vi "3.0.0_Power_Tunings & AW_Performance_Test_ECO_&_BOOST.vi"(6 ".bat":T1={"getVersion"="Getting Software Version.bat", "Start Test mode"="Start Test Mode.bat", "Start camera test mode"="Start camera test mode.bat", "get one RAW Image"="Get one image.bat", "Stop camera test mode"="Stop camera test mode.bat", "Stop Test Mode"="Stop Test Mode.bat", "Get image reflection"="Get image reflection.bat", "Get image uniformity andFlash LED brightness"="Get image uniformity andFlash LED brightness.bat", "Disable flash LED"="Disable flash LED.bat", "Enable flash LED"="Enable flash LED.bat", "Software Reset"="Software Reset.bat", "Tune Flash LED brightness"="Tune Flash LED brightness.bat", "Start Camera calibration"="Start Camera calibration.bat", "Verify OBC Setting"="Verify OBC Setting.bat"}, 7 "Data in":T2, 8 "error in (no error)":errorcluster, 9 "AllControls In":T3, 11 "Message Queue out":T4) -> (0 "error out":errorcluster, 1 "Flow":string, 3 "Message Queue Out":T4, 5 "Data out":T2)   [LabVIEW 2017]
uses:
  Depends/AMC/subVIs/TypeDefs/amc_Message Queue.ctl
  Depends/AMC/subVIs/TypeDefs/amc_Message.ctl
  Depends/Tools/Keyed Array/Tools_KeyedArray KeyedArray.ctl
  Ctrls/AllControls.ctl
  Ctrls/CSV_Data.ctl
  Ctrls/NFC.bat
panel:
  out "Unifority_Flag":bool
  out "Reflect_Flag":bool
  in  "Numeric 2":i32
  in  "Numeric":i32
types:
  T1 = typedef "NFC.bat" = cluster{"getVersion":string, "Start Test mode":string, "Start camera test mode":string, "get one RAW Image":string, "Stop camera test mode":string, "Stop Test Mode":string, "Get image reflection":string, "Get image uniformity andFlash LED brightness":string, "Disable flash LED":string, "Enable flash LED":string, "Software Reset":string, "Tune Flash LED brightness":string, "Start Camera calibration":string, "Verify OBC Setting":string}
  T2 = typedef "CSV_Data.ctl" = cluster{"Version":cluster{"SC_Version":string, "VP_Version":string}, "SN":string, "Table":string[][], "Count":cluster{"Total":i32, "OK":i32, "NG":i32, "Yield":dbl}, "Start Time":timestamp, "daemon reference":refnum<k5>, "CT":dbl, "Config":string[][], "OK/NG":bool, "Station ID":string, "MES DDM SN":string, "MES PCBA SN":string, "Retest":string, "Lux":string, "VOT":cluster{"Initial brightness":string, "Mean uniformity":string, "Uniformity_Deviation":string, "Adjusted brightness":string, "Mean_Adjusted":string, "Deviation_Adjusted":string, "Reflection":string, "Result":bool}, "SKU":string, "Plate_Diameter":string, "Alarm":string}
  T3 = typedef "AllControls.ctl" = cluster{"MainVI":refnum<vi>, "AlarmInfo":refnum<vi>, "Log":refnum<vi>, "Current CT":refnum<vi>, "ProductID":refnum<vi>, "Device state":refnum<vi>, "MES":refnum<vi>, "mode":refnum<vi>, "TestInfo":refnum<vi>, "SubPnl":refnum<vi>, "Table":refnum<vi>, "MES bool":refnum<vi>, "TestMode":refnum<vi>, "Recipe":refnum<vi>, "Fail resume":refnum<vi>, "LogIn":refnum<vi>, "Start":refnum<vi>, "Maintenance":refnum<vi>, "Stop":refnum<vi>, "Exit":refnum<vi>}
  T4 = typedef "amc_Message Queue.ctl" = refnum<queue>
  T5 = cluster{"getVersion":string, "Start Test mode":string, "Start camera test mode P1":string, "get one RAW Image":string, "Start camera test mode P0":string, "Stop Test Mode":string, "Stop Camera":string}
  T6 = typedef "HD Config.ctl" = cluster{" PC":cluster{"PC Address":u8[], "PC Port":i32}, "FCO":cluster{"COM":refnum<visa-resource-name>, "Baudrate":u32}, "DC Power ":cluster{"COM":refnum<visa-resource-name>, "Baudrate":u32}, "PW3336":cluster{"COM":refnum<visa-resource-name>, "Baudrate":u32}, "Lefoo":cluster{"COM":refnum<visa-resource-name>, "Baudrate":u32}, "Tempt&Hum":cluster{"COM":refnum<visa-resource-name>, "Baudrate":u32}, "DIPC":cluster{"COM":refnum<visa-resource-name>}, "Daemon":cluster{"IP Address":string, "Port":u16, "Retry":u16}, "NFC_Cmd":cluster{"COM":refnum<visa-resource-name>, "Baudrate":u32}, "Fail_resume_mode":bool, "GRR":bool, "NFC _Serial":cluster{"COM":refnum<visa-resource-name>, "Baudrate":u32}}
  T7 = typedef "Position Config.ctl" = cluster{"Black":dbl, "White":dbl, "Black1":dbl, "White1":dbl}
  T8 = typedef "TesterInfo.ctl" = cluster{"Station Name":string, "Station Code":string, "ES NO.":string, "Tester ID":string, "PassMark Revision":string, "Rig ID":string, "682_Tool_Repeat":string, "Project Name":string, "FFTesterPath":path, "Enable_User":bool, "Mode":enum16{"682"}, "Fail_resume_mode":bool}
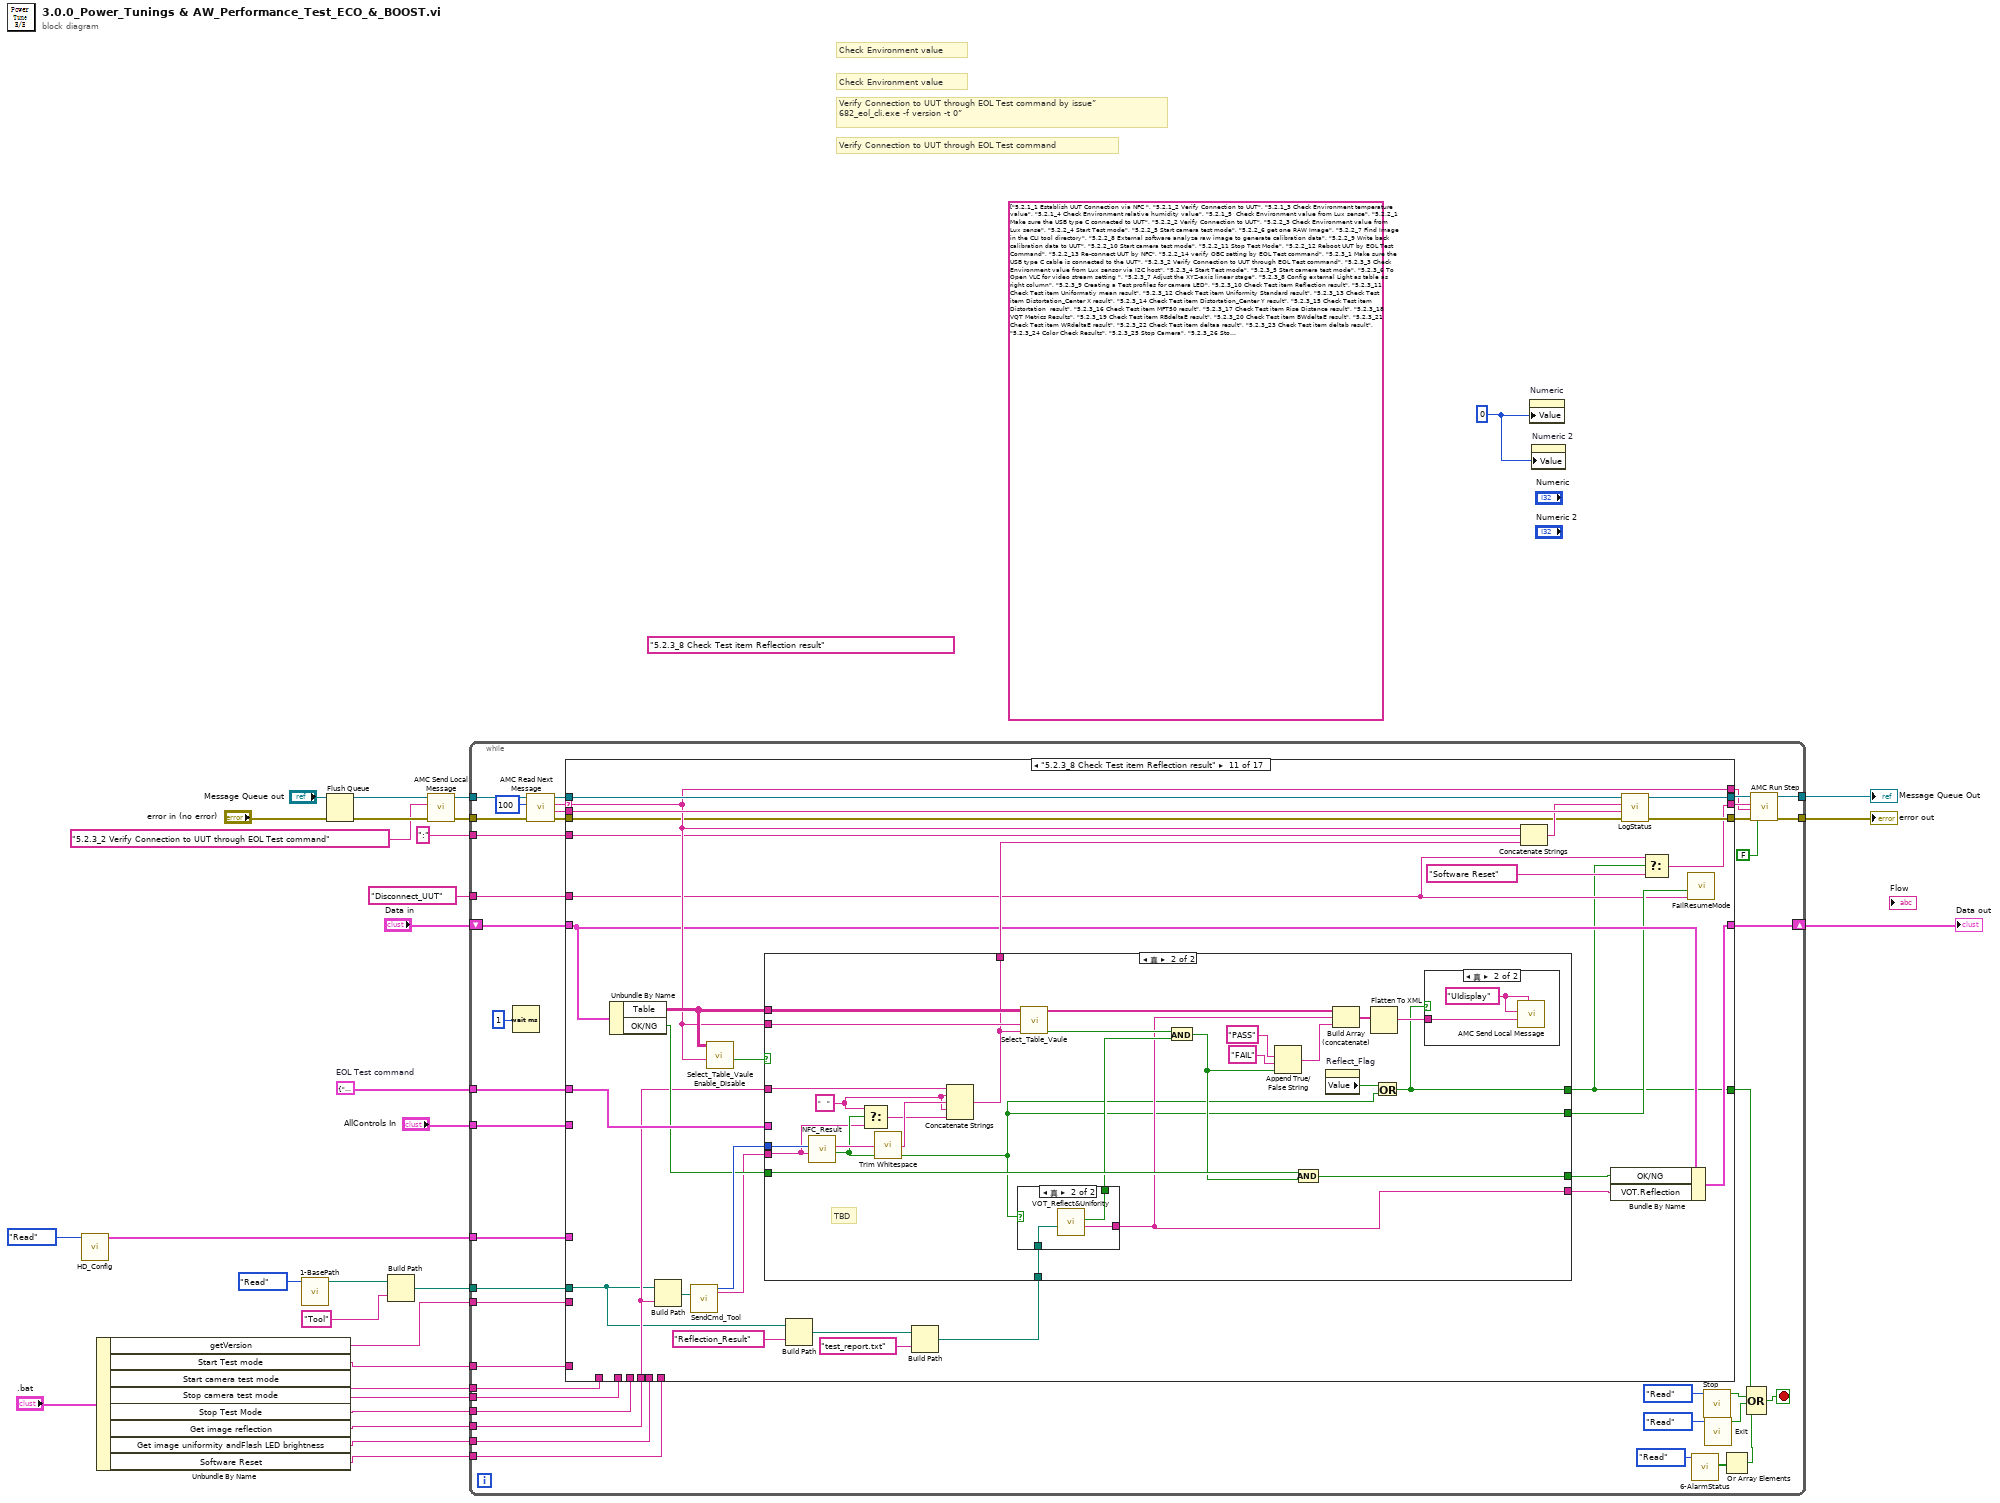
[diagram p0: block diagram]
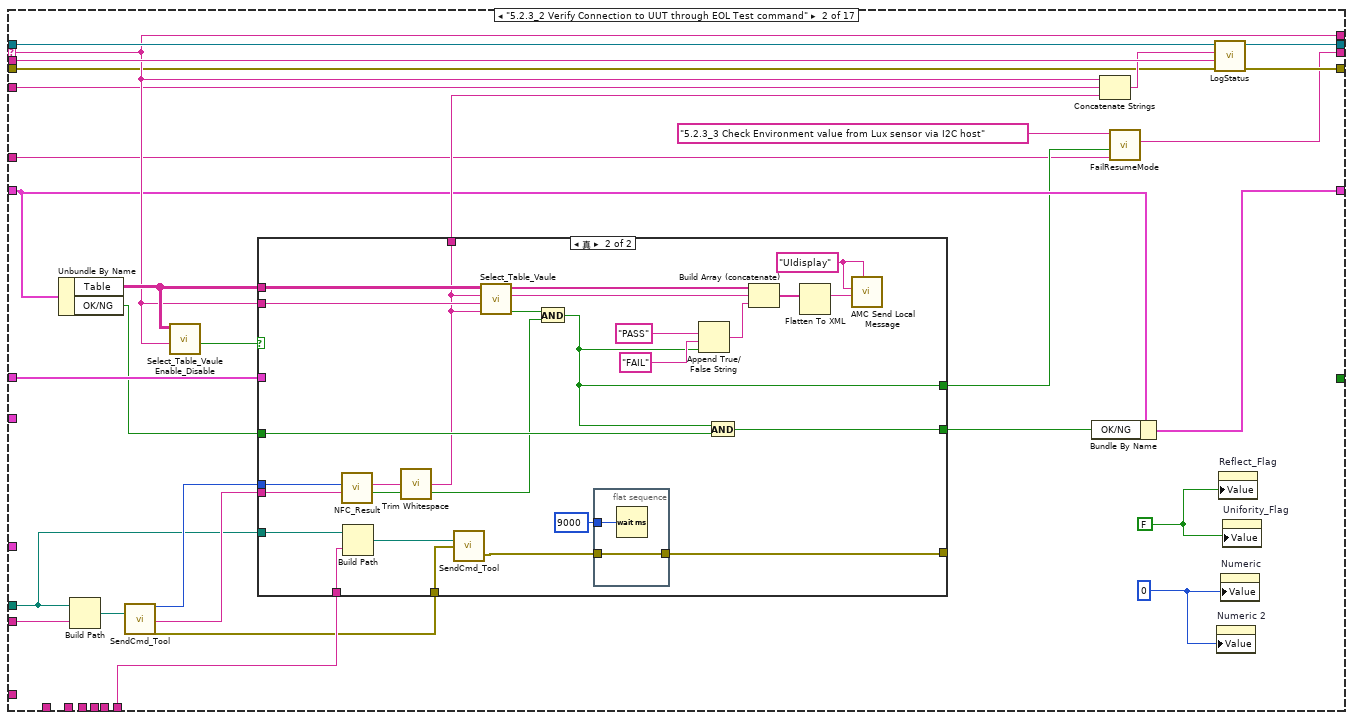
[diagram p3: hidden frame]
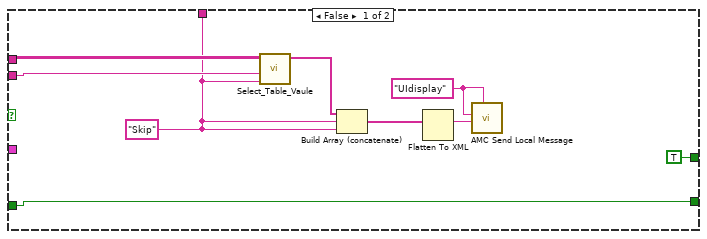
[diagram p4: hidden frame]
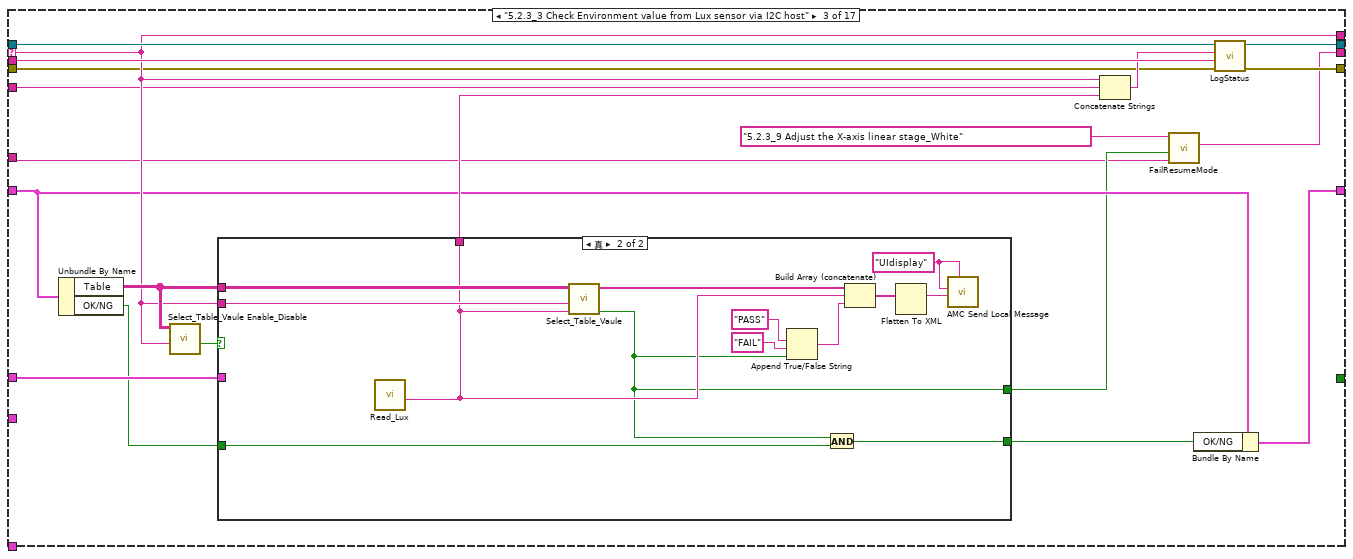
[diagram p5: hidden frame]
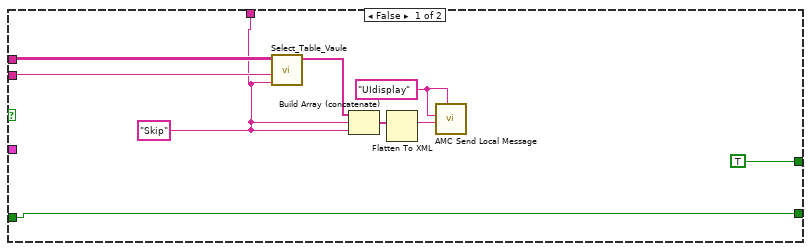
[diagram p6: hidden frame]
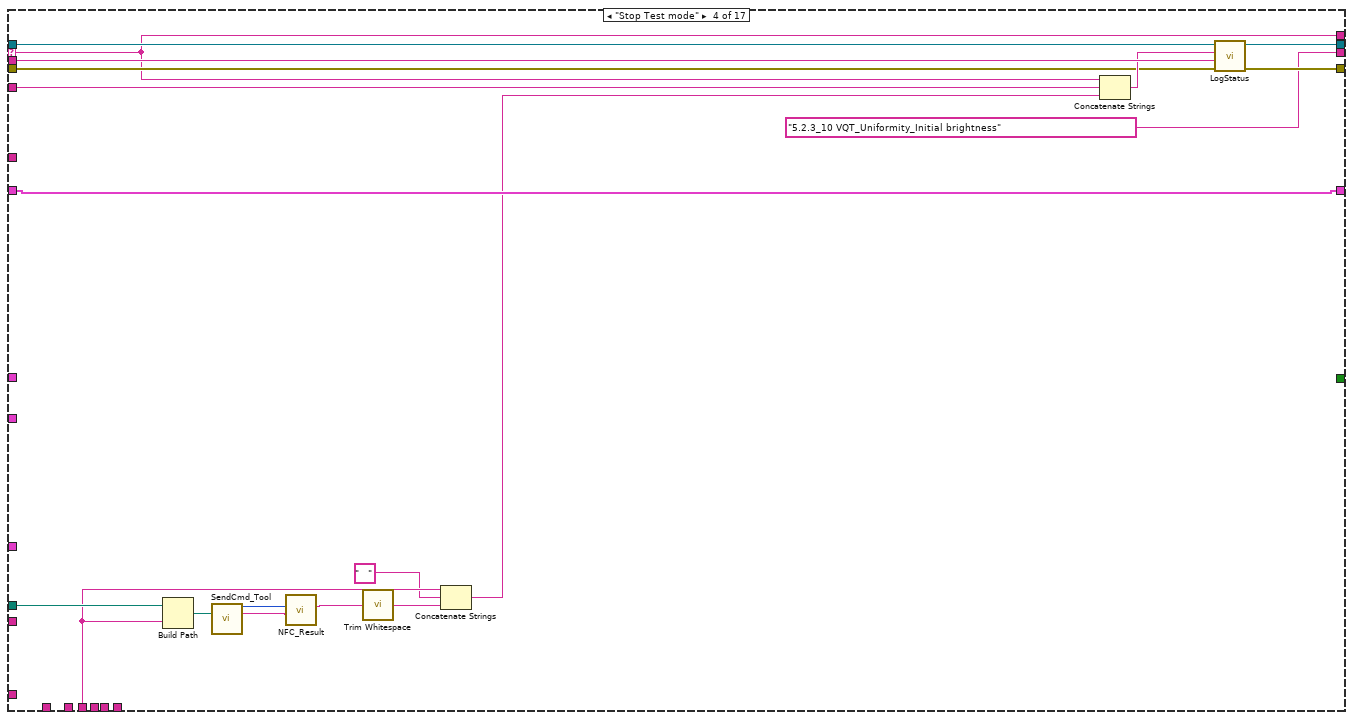
[diagram p7: hidden frame]
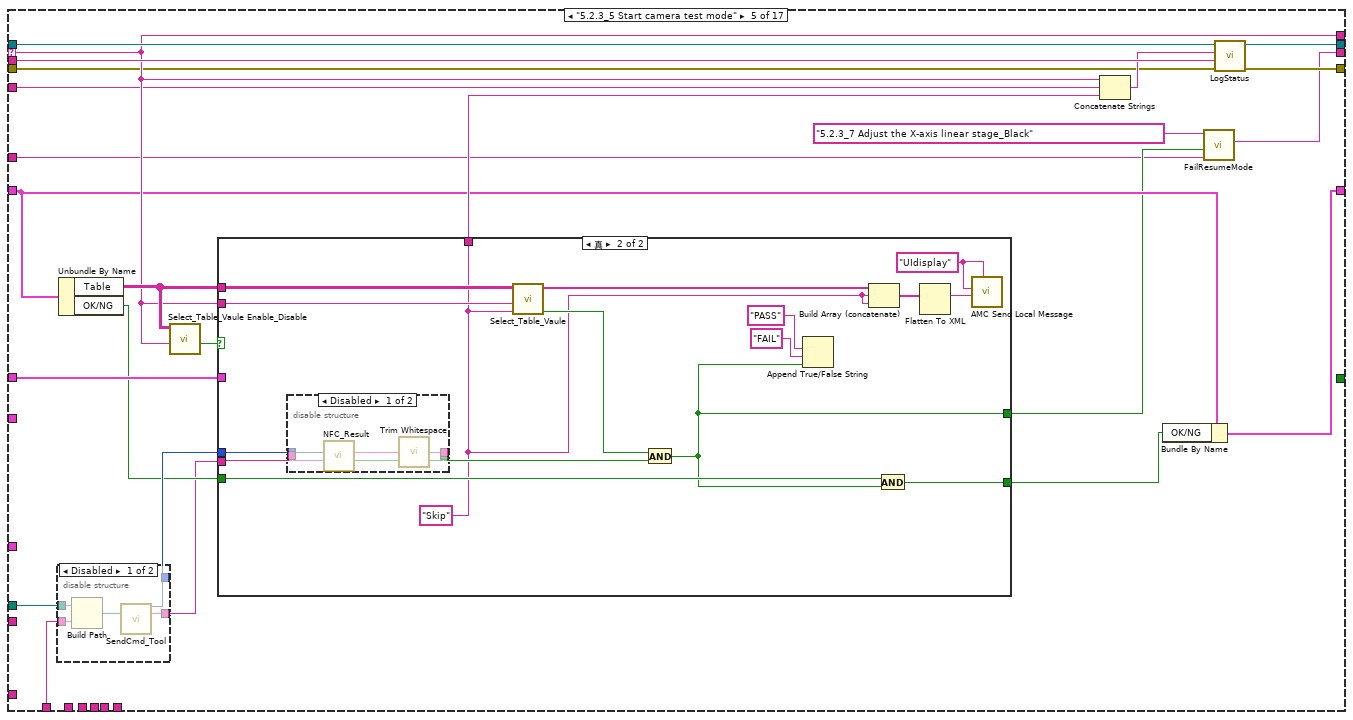
[diagram p8: hidden frame]
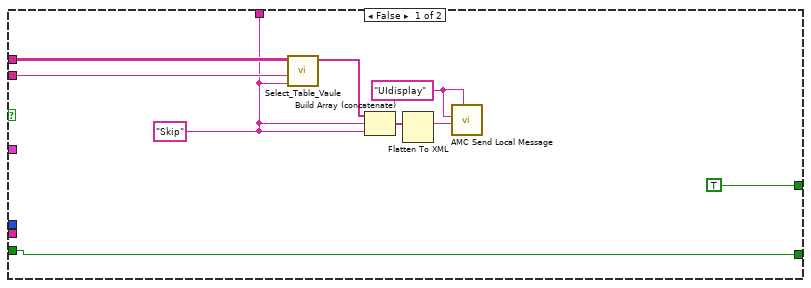
[diagram p10: hidden frame]
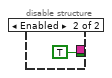
[diagram p11: hidden frame]
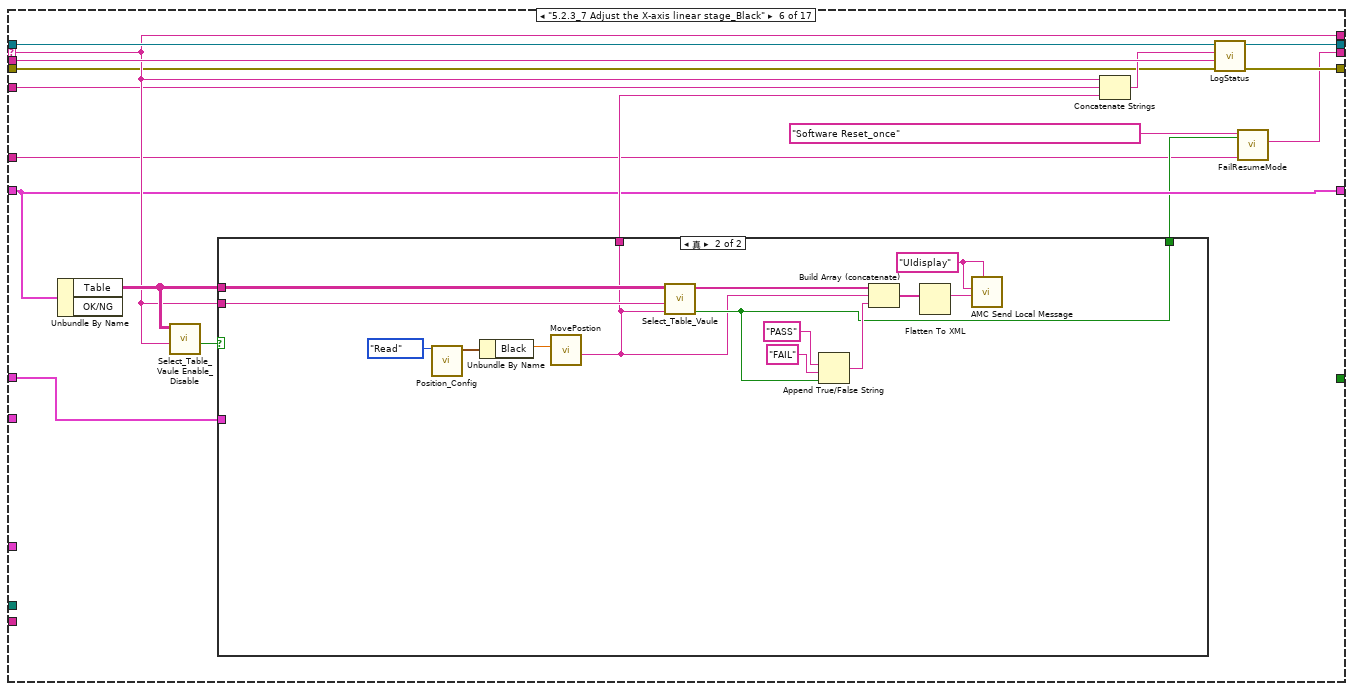
[diagram p12: hidden frame]
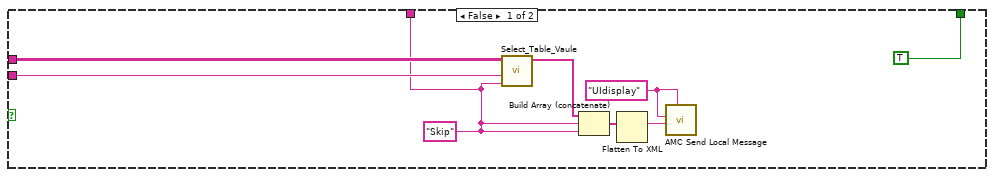
[diagram p13: hidden frame]
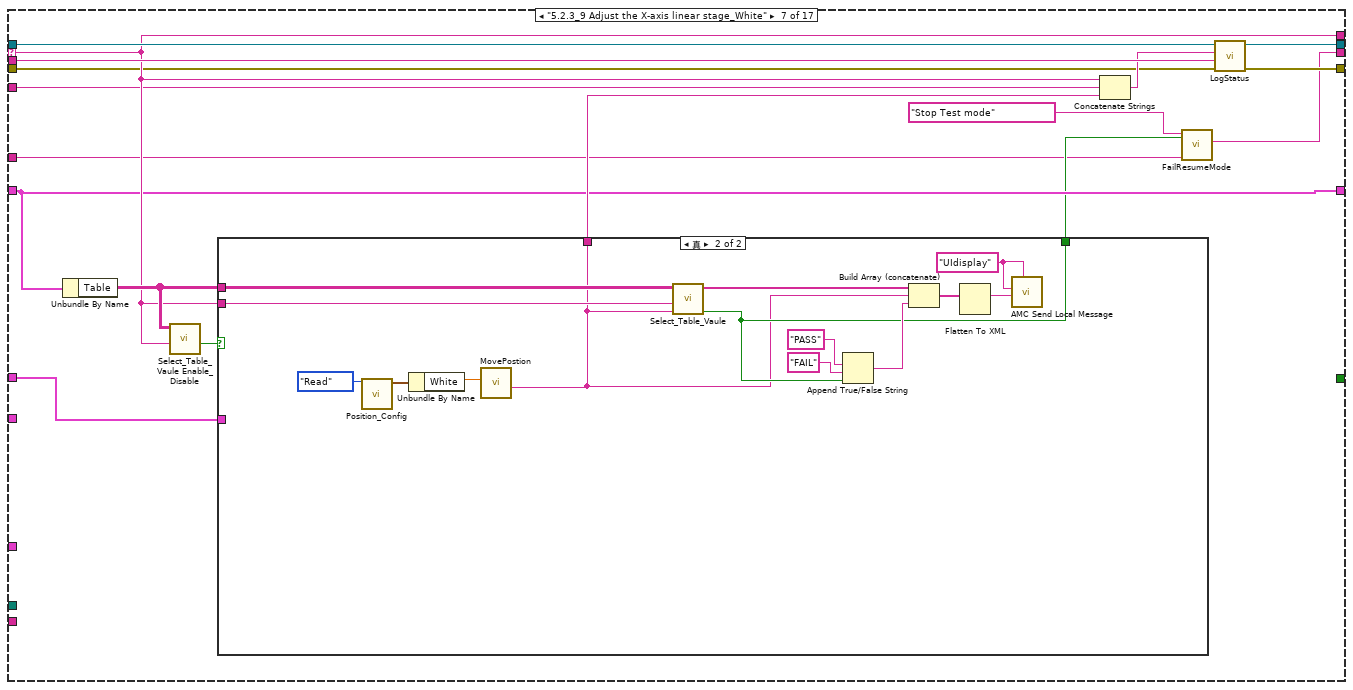
[diagram p14: hidden frame]
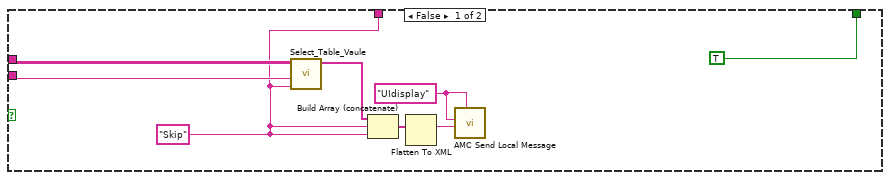
[diagram p15: hidden frame]
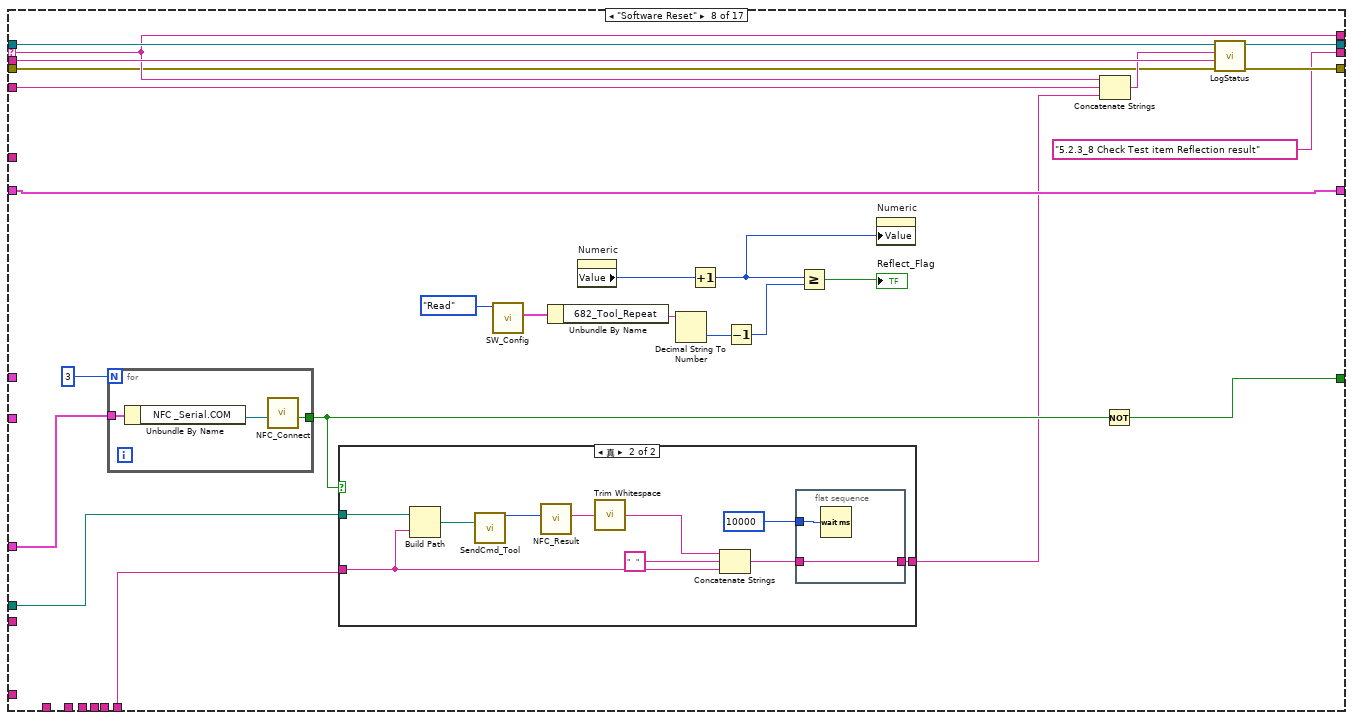
[diagram p16: hidden frame]
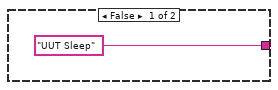
[diagram p17: hidden frame]
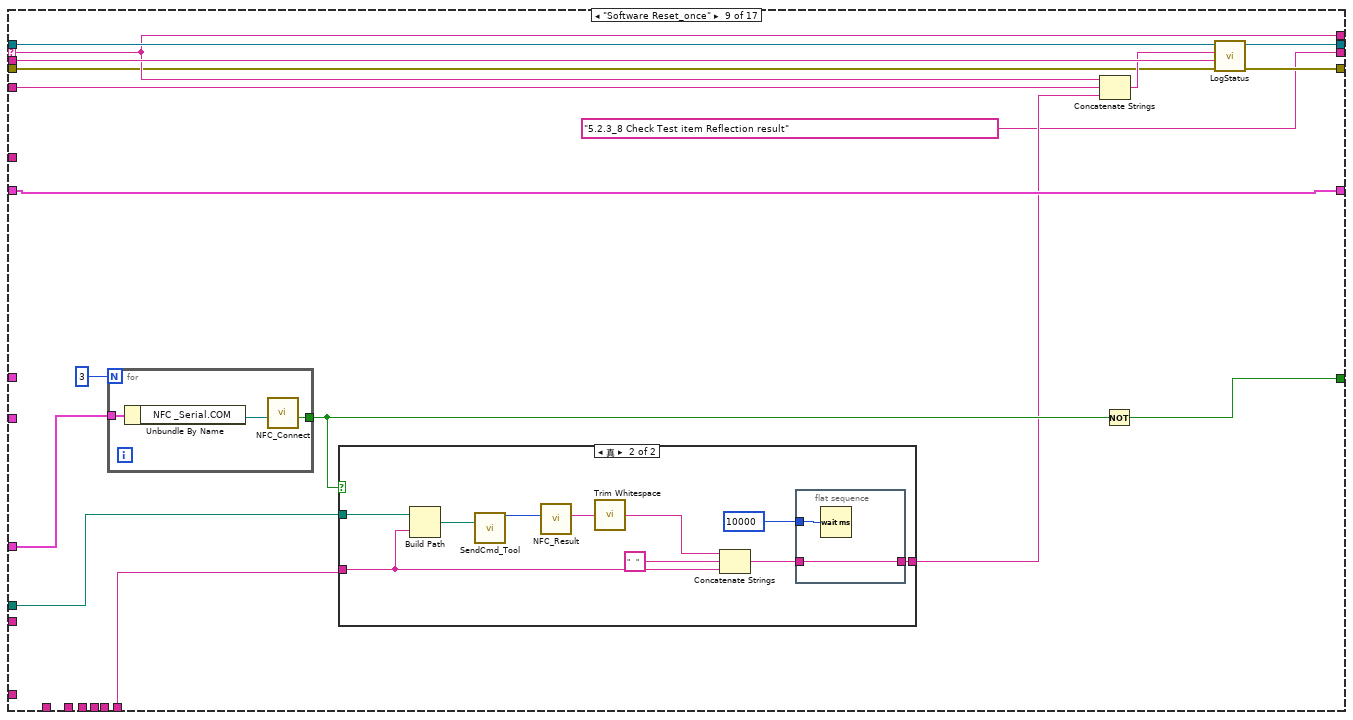
[diagram p18: hidden frame]
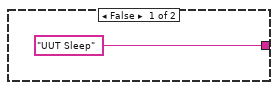
[diagram p19: hidden frame]
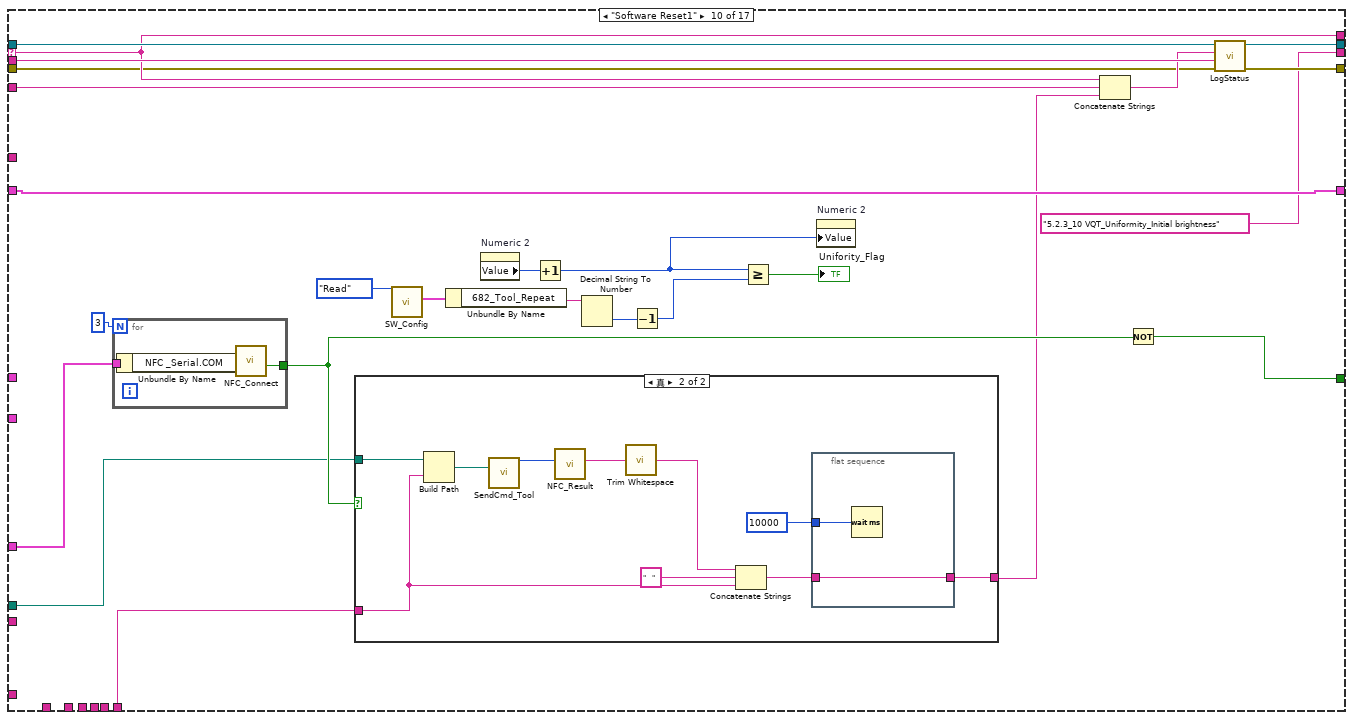
[diagram p20: hidden frame]
diagram:
  (unwired) "5.2.3_8 Check Test item Reflection result"
  w2 = 0 ("Numeric")
  (unwired) string[] ["5.2.1_1 Establish UUT Connection via NFC ", "5.2.1_2 Verify Connection to UUT", "5.2.1_3 Check Environment temperature value", "5.2.1_4 Check Environment relative humidity value", "5.2.1_5  Check Environment value from Lux sense", "5.2.2_1 Make sure the USB type C connected to UUT", "5.2.2_2 Verify Connection to UUT", "5.2.2_3 Check Environment value from Lux sense", "5.2.2_4 Start Test mode", "5.2.2_5 Start camera test mode", "5.2.2_6 get one RAW Image", "5.2.2_7 Find Image  in the CLI tool directory", "5.2.2_8 External software analyze raw image to generate calibration data", "5.2.2_9 Write back calibration data to UUT", "5.2.2_10 Start camera test mode", "5.2.2_11 Stop Test Mode", "5.2.2_12 Reboot UUT by EOL Test Command", "5.2.2_13 Re-connect UUT by NFC", "5.2.2_14 verify OBC setting by EOL Test command", "5.2.3_1 Make sure the USB type C cable is connected to the UUT", "5.2.3_2 Verify Connection to UUT through EOL Test command", "5.2.3_3 Check Environment value from Lux sensor via I2C host", "5.2.3_4 Start Test mode", "5.2.3_5 Start camera test mode", "5.2.3_6 To Open VLC for video stream setting ", "5.2.3_7 Adjust the XYZ-axis linear stage", "5.2.3_8 Config external Light as table as right column", "5.2.3_9 Creating a Test profiles for camera LED", "5.2.3_10 Check Test item Reflection result", "5.2.3_11 Check Test item Uniformatiy mean result", "5.2.3_12 Check Test item Uniformity Standard result", "5.2.3_13 Check Test item Distortation_Center X result", "5.2.3_14 Check Test item Distortation_Center Y result", "5.2.3_15 Check Test item Distortation  result", "5.2.3_16 Check Test item MFT50 result", "5.2.3_17 Check Test item Rise Distance result", "5.2.3_18 VQT Metrics Results", "5.2.3_19 Check Test item RBdeltaE result", "5.2.3_20 Check Test item BWdeltaE result", "5.2.3_21 Check Test item WRdeltaE result", "5.2.3_22 Check Test item deltaa result", "5.2.3_23 Check Test item deltab result", "5.2.3_24 Color Check Results", "5.2.3_25 Stop Camera", "5.2.3_26 Stop Test mode", "5.2.3_27 Shutdown UUT"] ("subarray")
  w17 = T5 {"getVersion"="682_eol_cli.exe -f version -t 0", "Start Test mode"="682_eol_cli.exe -f test -p 1", "Start camera test mode P1"="682_eol_cli.exe -f camera -p 1", "get one RAW Image"="“682_eol_cli.exe -f camera -p 2", "Start camera test mode P0"="682_eol_cli.exe -f camera -p 0", "Stop Test Mode"="682_eol_cli.exe -f test -p 0", "Stop Camera"="682_eol_cli.exe -f camera -p 0"}  # EOL Test command
  # "Check Environment value"
  # "Check Environment value"
  # "Verify Connection to UUT through EOL Test command by issue” \n682_eol_cli.exe -f version -t 0”"
  # "Verify Connection to UUT through EOL Test command"
  n1 = call "HD_Config.vi"("Step"=enum16{"Initial", "Write", "Read"}."Read") -> ("HD Config out"=w19:T6)  [unwired: 9 in, 1 out]
  n2 = Unbundle By Name(".bat") -> ("getVersion"=w12:string, "Start Test mode"=w11:string, "Start camera test mode"=w10:string, "Stop camera test mode"=w9:string, "Stop Test Mode"=w8:string, "Get image reflection"=w5:string, "Get image uniformity andFlash LED brightness"=w4:string, "Software Reset"=w3:string)
  n3 = call "1-BasePath.vi"("Step"=enum16{"Initial", "Write", "Read"}."Read") -> ("Path Out"=w14:path)  [unwired: 9 in, 1 out]
  n4 = Flush Queue(queue="Message Queue out") -> (queue out=w25:T4)  [unwired: 1 in, 2 out]
  n5 = Build Path(base path=w14, name or relative path="Tool") -> (appended path=w13:path)
  n6 = call "AMC Send Local Message.vi"("error in (no error)"="error in (no error)", "Message Name"="5.2.3_2 Verify Connection to UUT through EOL Test command", "Message Queue in"=w25) -> ("error out"=w28:errorcluster, "Message Queue out"=w29:T4)  [unwired: 7 in]
  n7 = while {
    tunnel: w29 -> [w70]
    tunnel: [w66] -> w24
    tunnel: w28 -> [w64]
    tunnel: [w61] -> w23
    tunnel: w19 -> [w58]
    shift-right: [w47] -> w21
    shift-left: "Data in" -> [w46]
    tunnel: "AllControls In" -> [w48]
    tunnel: w17 -> [w42]
    tunnel: w13 -> [w41]
    tunnel: w12 -> [w40]
    tunnel: w11 -> [w39]
    tunnel: w10 -> [w38]
    tunnel: w9 -> [w37]
    tunnel: w8 -> [w36]
    tunnel: ":" -> [w35]
    tunnel: "Disconnect_UUT" -> [w34]
    tunnel: w5 -> [w33]
    tunnel: w4 -> [w32]
    tunnel: w3 -> [w31]
    stop <- w49 stop-if-true
    n8 = Wait (ms)(milliseconds to wait=u32 1 ("等待时间（毫秒）")) -> ()  [unwired: 1 out]
    n9 = call "AMC Read Next Message.vi"("error in (no error)"=w64, "timeout (1ms)"=100, "Message Queue in"=w70) -> ("error out"=w63:errorcluster, "Message Value"=w56:string, "Message Name"=w68:string, "Message Queue out"=w69:T4)  [unwired: 1 in, 4 out]
    n10 = case shown="\"5.2.3_8 Check Test item Reflection result\"" w68 {
      selector: w68 -> [_ w95 w150 w182 w213 w265 w303 w351 w383 w423 w467 w544 w611 w652 w693 w734 w775]
      tunnel: w69 -> [w73 w101 w156 w196 w219 w271 w309 w355 w387 w427 w473 w550 w617 w658 w699 w740 w781]
      tunnel: [w73 w101 w156 w196 w219 w271 w309 w355 w387 w427 w473 w550 w617 w658 w699 w740 w781] -> w67
      tunnel: w63 -> [w72 w89 w143 w190 w208 w258 w296 w349 w381 w421 w464 w541 w608 w649 w690 w731 w772]
      tunnel: [w72 w100 w155 w195 w218 w270 w308 w354 w386 w426 w472 w549 w616 w657 w698 w739 w780] -> w62
      tunnel: [_ _ _ _ _ _ _ w338 w373 w412 w444 _ _ _ _ _ _] -> w50
      tunnel: w56 -> [_ w99 w154 w194 w217 w269 w307 w353 w385 w425 w471 w548 w615 w656 w697 w738 w779]
      tunnel: [_ w95 w150 w182 w213 w265 w303 w351 w383 w423 w467 w544 w611 w652 w693 w734 w775] -> w55
      tunnel: w58 -> [_ _ _ _ _ _ _ w344 w377 w416 _ _ _ _ _ _ _]
      tunnel: [_ w79 w139 "5.2.3_10 VQT_Uniformity_Initial brightness" w198 w256 w294 "5.2.3_8 Check Test item Reflection result" "5.2.3_8 Check Test item Reflection result" "5.2.3_10 VQT_Uniformity_Initial brightness" w446 w515 "5.2.3_12 VQT_Uniformity_Deviation" "5.2.3_13 VQT_Uniformity_Adjusted brightness" "5.2.3_14 VQT_Uniformity_Mean uniformity" "5.2.3_15 VQT_Uniformity_Deviation" "5.2.3_7 Adjust the X-axis linear stage_Black"] -> w57
      tunnel: w48 -> [_ _ _ _ _ _ _ _ _ _ _ _ _ _ _ _ _]
      tunnel: [w71 w85 w146 w185 w203 w263 w301 w350 w382 w422 w457 w533 w603 w644 w685 w726 w767] -> w47
      tunnel: w46 -> [w71 w88 w147 w185 w205 w263 w301 w350 w382 w422 w459 w534 w605 w646 w687 w728 w769]
      tunnel: w42 -> [_ w93 w148 _ w211 w262 w300 _ _ _ w465 w542 w609 w650 w691 w732 w773]
      tunnel: w41 -> [_ w78 _ w192 w210 _ _ w343 w376 w415 w452 w524 _ _ _ _ _]
      tunnel: w40 -> [_ w92 _ _ _ _ _ _ _ _ _ _ _ _ _ _ _]
      tunnel: w39 -> [_ _ _ _ _ _ _ _ _ _ _ _ _ _ _ _ _]
      tunnel: w38 -> [_ _ _ _ w209 _ _ _ _ _ _ _ _ _ _ _ _]
      tunnel: w37 -> [_ _ _ _ _ _ _ _ _ _ _ _ _ _ _ _ _]
      tunnel: w36 -> [_ _ _ w186 _ _ _ _ _ _ _ _ _ _ _ _ _]
      tunnel: w35 -> [_ w83 w142 w188 w201 w261 w299 w348 w380 w420 w463 w540 w607 w648 w689 w730 w771]
      tunnel: w34 -> [_ w80 w140 _ w197 w259 w297 _ _ _ w445 w539 _ _ _ _ _]
      tunnel: w33 -> [_ _ _ _ _ _ _ _ _ _ w456 _ _ _ _ _ _]
      tunnel: w32 -> [_ _ _ _ _ _ _ _ _ _ _ w528 _ _ _ _ _]
      tunnel: w31 -> [_ w77 _ _ _ _ _ w342 w375 w414 _ _ _ _ _ _ _]
      frame "假", Default {
      }
      frame "5.2.3_2 Verify Connection to UUT through EOL Test command" {
        w74 = FALSE ("2")
        w75 = 0 ("Numeric")
        n11 = Unbundle By Name(w88) -> ("Table"=w96:string[][], "OK/NG"=w87:bool)
        n12 = Build Path(base path=w78, name or relative path=w92) -> (appended path=w91:path)
        n13 = call "SendCmd_Tool.vi"("path_bat"=w91) -> ("return code"=w90:i32, "error out 3"=w76:errorcluster, "version info"=w84:string)  [unwired: 7 in, 5 out]
        n14 = call "Select_Table_Vaule Enable_Disable.vi"("Action"=w95, "Table"=w96) -> ("Enable"=w94:bool)  [unwired: 8 in, 1 out]
        n15 = case shown="真" w94 {
          tunnel: [w103 w123] -> w97
          tunnel: w96 -> [w105 w129]
          tunnel: w95 -> [w104 w128]
          tunnel: w93 -> [_ _]
          tunnel: w90 -> [_ w122]
          tunnel: w87 -> [w102 w125]
          tunnel: [w102 w124] -> w86
          tunnel: w84 -> [_ w119]
          tunnel: [TRUE w118] -> w81
          tunnel: w78 -> [_ w116]
          tunnel: w77 -> [_ w115]
          tunnel: w76 -> [_ w114]
          tunnel: [_ w111] -> _
          frame False {
            w109 = "UIdisplay" ("Process (\"\" - local)")
            w103 = "Skip" ("Action")
            n16 = call "Select_Table_Vaule.vi"("Vaule"=w103, "Action"=w104, "Table"=w105) -> ("vaule"=w106:string[])  [unwired: 7 in, 1 out]
            n17 = Build Array (concatenate)(w106, w103, w103) -> (w108:string[])
            n18 = Flatten To XML(anything=w108) -> (xml string=w107:string)
            n19 = call "AMC Send Local Message.vi"("Process (\"\" - local)"=w109, "Message Value"=w107, "Message Name"=w109) -> ()  [unwired: 7 in, 2 out]
          }
          frame True {
            w134 = "UIdisplay" ("Process (\"\" - local)")
            n20 = call "NFC_Result.vi"("input"=w119, "return code"=w122) -> ("Command Sucess"=w121:bool, "return_result"=w120:string)  [unwired: 8 in]
            n21 = Build Path(base path=w116, name or relative path=w115) -> (appended path=w117:path)
            n22 = call <vilib>:"Trim Whitespace.vi"("string"=w120) -> ("trimmed string"=w123:string)  [unwired: 1 in]
            n23 = call "SendCmd_Tool.vi"("path_bat"=w117, "error in (no error) 2"=w114) -> ("error out 3"=w112:errorcluster)  [unwired: 6 in, 7 out]
            n24 = call "Select_Table_Vaule.vi"("Vaule"=w123, "Action"=w128, "Table"=w129) -> ("Result"=w126:bool, "vaule"=w135:string[])  [unwired: 7 in]
            n25 = And(x=w126, y=w121) -> (x .and. y?=w118:bool)
            n26 = flat-sequence {
              tunnel: u32 9000 ("milliseconds to wait") -> [w137]
              tunnel: w112 -> [w136]
              tunnel: [w136] -> w111
              frame #0 {
                n27 = Wait (ms)(milliseconds to wait=w137) -> ()  [unwired: 1 out]
              }
            }
            n28 = Append True/False String(1:w118, 2:"FAIL" ("真字符串"), 3:"PASS" ("真字符串")) -> (0:w127:string)  [unwired: 1 in]
            n29 = And(x=w118, y=w125) -> (x .and. y?=w124:bool)
            n30 = Build Array (concatenate)(w135, w123, w127) -> (w133:string[])
            n31 = Flatten To XML(anything=w133) -> (xml string=w132:string)
            n32 = call "AMC Send Local Message.vi"("Process (\"\" - local)"=w134, "Message Value"=w132, "Message Name"=w134) -> ()  [unwired: 7 in, 2 out]
          }
        }
        n33 = Bundle By Name(cluster=w88, "OK/NG"=w86) -> (w85:T2)
        n34 = Concatenate Strings(w95, w83, w97) -> (w98:string)
        n35 = call "FailResumeMode.vi"("NextMessage"="5.2.3_3 Check Environment value from Lux sensor via I2C host", "OK/NG"=w81, "EndMessage"=w80) -> ("OutMessage"=w79:string)  [unwired: 6 in]
        n36 = call "LogStatus.vi"("error in (no error)"=w89, "last message"=w99, "message"=w98) -> ("error  out"=w100:errorcluster)  [unwired: 8 in]
        n37 = property on="Numeric 2" class="DigNum (严格)"("Value"=w75) -> ()  [unwired: 2 in, 2 out]
        n38 = property on="Reflect_Flag" class="Bool (严格)"("Value"=w74) -> ()  [unwired: 2 in, 2 out]
        n39 = property on="Numeric" class="DigNum (严格)"("Value"=w75) -> ()  [unwired: 2 in, 2 out]
        n40 = property on="Unifority_Flag" class="Bool (严格)"("Value"=w74) -> ()  [unwired: 2 in, 2 out]
      }
      frame "5.2.3_3 Check Environment value from Lux sensor via I2C host" {
        n41 = Unbundle By Name(w147) -> ("Table"=w151:string[][], "OK/NG"=w145:bool)
        n42 = call "Select_Table_Vaule Enable_Disable.vi"("Action"=w150, "Table"=w151) -> ("Enable"=w149:bool)  [unwired: 8 in, 1 out]
        n43 = case shown="真" w149 {
          tunnel: [w158 w169] -> w152
          tunnel: w151 -> [w160 w172]
          tunnel: w150 -> [w159 w171]
          tunnel: w148 -> [_ _]
          tunnel: w145 -> [w157 w168]
          tunnel: [w157 w167] -> w144
          tunnel: [TRUE ("Result") w166] -> w141
          frame False {
            w164 = "UIdisplay" ("Process (\"\" - local)")
            w158 = "Skip" ("Action")
            n44 = call "Select_Table_Vaule.vi"("Vaule"=w158, "Action"=w159, "Table"=w160) -> ("vaule"=w161:string[])  [unwired: 7 in, 1 out]
            n45 = Build Array (concatenate)(w161, w158, w158) -> (w163:string[])
            n46 = Flatten To XML(anything=w163) -> (xml string=w162:string)
            n47 = call "AMC Send Local Message.vi"("Process (\"\" - local)"=w164, "Message Value"=w162, "Message Name"=w164) -> ()  [unwired: 7 in, 2 out]
          }
          frame True {
            w177 = "UIdisplay" ("Process (\"\" - local)")
            n48 = call "Read_Lux.vi"() -> ("Lux_Value"=w169:string)  [unwired: 9 in, 2 out]
            n49 = call "Select_Table_Vaule.vi"("Vaule"=w169, "Action"=w171, "Table"=w172) -> ("Result"=w166:bool, "vaule"=w178:string[])  [unwired: 7 in]
            n50 = Append True/False String(1:w166, 2:"FAIL" ("真字符串"), 3:"PASS" ("真字符串")) -> (0:w170:string)  [unwired: 1 in]
            n51 = And(x=w166, y=w168) -> (x .and. y?=w167:bool)
            n52 = Build Array (concatenate)(w178, w169, w170) -> (w176:string[])
            n53 = Flatten To XML(anything=w176) -> (xml string=w175:string)
            n54 = call "AMC Send Local Message.vi"("Process (\"\" - local)"=w177, "Message Value"=w175, "Message Name"=w177) -> ()  [unwired: 7 in, 2 out]
          }
        }
        n55 = Concatenate Strings(w150, w142, w152) -> (w153:string)
        n56 = call "FailResumeMode.vi"("NextMessage"="5.2.3_9 Adjust the X-axis linear stage_White", "OK/NG"=w141, "EndMessage"=w140) -> ("OutMessage"=w139:string)  [unwired: 6 in]
        n57 = Bundle By Name(cluster=w147, "OK/NG"=w144) -> (w146:T2)
        n58 = call "LogStatus.vi"("error in (no error)"=w143, "last message"=w154, "message"=w153) -> ("error  out"=w155:errorcluster)  [unwired: 8 in]
      }
      frame "Stop Test mode" {
        n59 = Build Path(base path=w192, name or relative path=w186) -> (appended path=w187:path)
        n60 = call "SendCmd_Tool.vi"("path_bat"=w187) -> ("return code"=w191:i32, "Other"=w189:string)  [unwired: 7 in, 6 out]
        n61 = call "NFC_Result.vi"("input"=w189, "return code"=w191) -> ("return_result"=w184:string)  [unwired: 8 in, 1 out]
        n62 = call <vilib>:"Trim Whitespace.vi"("string"=w184) -> ("trimmed string"=w181:string)  [unwired: 1 in]
        n63 = Concatenate Strings(w186, "   ", w181) -> (w180:string)
        n64 = Concatenate Strings(w182, w188, w180) -> (w193:string)
        n65 = call "LogStatus.vi"("error in (no error)"=w190, "last message"=w194, "message"=w193) -> ("error  out"=w195:errorcluster)  [unwired: 8 in]
      }
      frame "5.2.3_5 Start camera test mode" {
        n66 = disable-structure shown="Disabled" {
          disable-tunnel: w210 -> [w223 _]
          disable-tunnel: w209 -> [w222 _]
          disable-tunnel: [w221 _] -> w207
          disable-tunnel: [w220 _] -> w202
          frame Disabled {
            n67 = Build Path(base path=w223, name or relative path=w222) -> (appended path=w224:path)
            n68 = call "SendCmd_Tool.vi"("path_bat"=w224) -> ("return code"=w221:i32, "Other"=w220:string)  [unwired: 7 in, 6 out]
          }
          frame Enabled {
          }
        }
        n69 = Unbundle By Name(w205) -> ("Table"=w214:string[][], "OK/NG"=w206:bool)
        n70 = call "Select_Table_Vaule Enable_Disable.vi"("Action"=w213, "Table"=w214) -> ("Enable"=w212:bool)  [unwired: 8 in, 1 out]
        n71 = case shown="真" w212 {
          tunnel: [w226 w234] -> w215
          tunnel: w214 -> [w228 w243]
          tunnel: w213 -> [w227 w242]
          tunnel: w211 -> [_ _]
          tunnel: w207 -> [_ w238]
          tunnel: w206 -> [w225 w240]
          tunnel: [w225 w239] -> w204
          tunnel: w202 -> [_ w236]
          tunnel: [TRUE w235] -> w199
          frame False {
            w232 = "UIdisplay" ("Process (\"\" - local)")
            w226 = "Skip" ("Action")
            n72 = call "Select_Table_Vaule.vi"("Vaule"=w226, "Action"=w227, "Table"=w228) -> ("vaule"=w229:string[])  [unwired: 7 in, 1 out]
            n73 = Build Array (concatenate)(w229, w226, w226) -> (w231:string[])
            n74 = Flatten To XML(anything=w231) -> (xml string=w230:string)
            n75 = call "AMC Send Local Message.vi"("Process (\"\" - local)"=w232, "Message Value"=w230, "Message Name"=w232) -> ()  [unwired: 7 in, 2 out]
          }
          frame True {
            w234 = "Skip" ("response")
            w248 = "UIdisplay" ("Process (\"\" - local)")
            n76 = disable-structure shown="Disabled" {
              disable-tunnel: w238 -> [w254 _]
              disable-tunnel: [w253 TRUE ("Command Sucess")] -> w237
              disable-tunnel: w236 -> [w251 _]
              disable-tunnel: [w250 _] -> _
              frame Disabled {
                n77 = call "NFC_Result.vi"("input"=w251, "return code"=w254) -> ("Command Sucess"=w253:bool, "return_result"=w252:string)  [unwired: 8 in]
                n78 = call <vilib>:"Trim Whitespace.vi"("string"=w252) -> ("trimmed string"=w250:string)  [unwired: 1 in]
              }
              frame Enabled {
              }
            }
            n79 = call "Select_Table_Vaule.vi"("Vaule"=w234, "Action"=w242, "Table"=w243) -> ("Result"=w241:bool, "vaule"=w249:string[])  [unwired: 7 in]
            n80 = And(x=w241, y=w237) -> (x .and. y?=w235:bool)
            n81 = Append True/False String(1:w235, 2:"FAIL" ("真字符串"), 3:"PASS" ("真字符串")) -> ()  [unwired: 1 in, 1 out]
            n82 = Build Array (concatenate)(w249, w234, w234) -> (w247:string[])
            n83 = And(x=w240, y=w235) -> (x .and. y?=w239:bool)
            n84 = Flatten To XML(anything=w247) -> (xml string=w246:string)
            n85 = call "AMC Send Local Message.vi"("Process (\"\" - local)"=w248, "Message Value"=w246, "Message Name"=w248) -> ()  [unwired: 7 in, 2 out]
          }
        }
        n86 = Concatenate Strings(w213, w201, w215) -> (w216:string)
        n87 = Bundle By Name(cluster=w205, "OK/NG"=w204) -> (w203:T2)
        n88 = call "FailResumeMode.vi"("NextMessage"="5.2.3_7 Adjust the X-axis linear stage_Black", "OK/NG"=w199, "EndMessage"=w197) -> ("OutMessage"=w198:string)  [unwired: 6 in]
        n89 = call "LogStatus.vi"("error in (no error)"=w208, "last message"=w217, "message"=w216) -> ("error  out"=w218:errorcluster)  [unwired: 8 in]
      }
      frame "5.2.3_7 Adjust the X-axis linear stage_Black" {
        n90 = Unbundle By Name(w263) -> ("Table"=w266:string[][])  [unwired: 1 out]
        n91 = call "Select_Table_Vaule Enable_Disable.vi"("Action"=w265, "Table"=w266) -> ("Enable"=w264:bool)  [unwired: 8 in, 1 out]
        n92 = case shown="真" w264 {
          tunnel: [w272 w280] -> w267
          tunnel: w266 -> [w274 w287]
          tunnel: w265 -> [w273 w286]
          tunnel: w262 -> [_ _]
          tunnel: [TRUE ("Result") w284] -> w260
          frame False {
            w278 = "UIdisplay" ("Process (\"\" - local)")
            w272 = "Skip" ("Action")
            n93 = call "Select_Table_Vaule.vi"("Vaule"=w272, "Action"=w273, "Table"=w274) -> ("vaule"=w275:string[])  [unwired: 7 in, 1 out]
            n94 = Build Array (concatenate)(w275, w272, w272) -> (w277:string[])
            n95 = Flatten To XML(anything=w277) -> (xml string=w276:string)
            n96 = call "AMC Send Local Message.vi"("Process (\"\" - local)"=w278, "Message Value"=w276, "Message Name"=w278) -> ()  [unwired: 7 in, 2 out]
          }
          frame True {
            w292 = "UIdisplay" ("Process (\"\" - local)")
            n97 = call "Position_Config.vi"("Step"=enum16{"Initial", "Write", "Read"}."Read") -> ("Position Config out"=w282:T7)  [unwired: 9 in, 1 out]
            n98 = Unbundle By Name(w282) -> ("Black"=w281:dbl)
            n99 = call "MovePostion.vi"("position"=w281) -> ("MoveDisance"=w280:string)  [unwired: 9 in, 1 out]
            n100 = call "Select_Table_Vaule.vi"("Vaule"=w280, "Action"=w286, "Table"=w287) -> ("Result"=w284:bool, "vaule"=w293:string[])  [unwired: 7 in]
            n101 = Append True/False String(1:w284, 2:"FAIL" ("真字符串"), 3:"PASS" ("真字符串")) -> (0:w285:string)  [unwired: 1 in]
            n102 = Build Array (concatenate)(w293, w280, w285) -> (w291:string[])
            n103 = Flatten To XML(anything=w291) -> (xml string=w290:string)
            n104 = call "AMC Send Local Message.vi"("Process (\"\" - local)"=w292, "Message Value"=w290, "Message Name"=w292) -> ()  [unwired: 7 in, 2 out]
          }
        }
        n105 = Concatenate Strings(w265, w261, w267) -> (w268:string)
        n106 = call "LogStatus.vi"("error in (no error)"=w258, "last message"=w269, "message"=w268) -> ("error  out"=w270:errorcluster)  [unwired: 8 in]
        n107 = call "FailResumeMode.vi"("NextMessage"="Software Reset_once", "OK/NG"=w260, "EndMessage"=w259) -> ("OutMessage"=w256:string)  [unwired: 6 in]
      }
      frame "5.2.3_9 Adjust the X-axis linear stage_White" {
        n108 = Unbundle By Name(w301) -> ("Table"=w304:string[][])
        n109 = call "Select_Table_Vaule Enable_Disable.vi"("Action"=w303, "Table"=w304) -> ("Enable"=w302:bool)  [unwired: 8 in, 1 out]
        n110 = case shown="真" w302 {
          tunnel: [w310 w318] -> w305
          tunnel: w304 -> [w312 w325]
          tunnel: w303 -> [w311 w324]
          tunnel: w300 -> [_ _]
          tunnel: [TRUE ("Result") w322] -> w298
          frame False {
            w316 = "UIdisplay" ("Process (\"\" - local)")
            w310 = "Skip" ("Action")
            n111 = call "Select_Table_Vaule.vi"("Vaule"=w310, "Action"=w311, "Table"=w312) -> ("vaule"=w313:string[])  [unwired: 7 in, 1 out]
            n112 = Build Array (concatenate)(w313, w310, w310) -> (w315:string[])
            n113 = Flatten To XML(anything=w315) -> (xml string=w314:string)
            n114 = call "AMC Send Local Message.vi"("Process (\"\" - local)"=w316, "Message Value"=w314, "Message Name"=w316) -> ()  [unwired: 7 in, 2 out]
          }
          frame True {
            w330 = "UIdisplay" ("Process (\"\" - local)")
            n115 = call "Position_Config.vi"("Step"=enum16{"Initial", "Write", "Read"}."Read") -> ("Position Config out"=w320:T7)  [unwired: 9 in, 1 out]
            n116 = Unbundle By Name(w320) -> ("White"=w319:dbl)
            n117 = call "MovePostion.vi"("position"=w319) -> ("MoveDisance"=w318:string)  [unwired: 9 in, 1 out]
            n118 = call "Select_Table_Vaule.vi"("Vaule"=w318, "Action"=w324, "Table"=w325) -> ("Result"=w322:bool, "vaule"=w331:string[])  [unwired: 7 in]
            n119 = Append True/False String(1:w322, 2:"FAIL" ("真字符串"), 3:"PASS" ("真字符串")) -> (0:w323:string)  [unwired: 1 in]
            n120 = Build Array (concatenate)(w331, w318, w323) -> (w329:string[])
            n121 = Flatten To XML(anything=w329) -> (xml string=w328:string)
            n122 = call "AMC Send Local Message.vi"("Process (\"\" - local)"=w330, "Message Value"=w328, "Message Name"=w330) -> ()  [unwired: 7 in, 2 out]
          }
        }
        n123 = Concatenate Strings(w303, w299, w305) -> (w306:string)
        n124 = call "FailResumeMode.vi"("NextMessage"="Stop Test mode", "OK/NG"=w298, "EndMessage"=w297) -> ("OutMessage"=w294:string)  [unwired: 6 in]
        n125 = call "LogStatus.vi"("error in (no error)"=w296, "last message"=w307, "message"=w306) -> ("error  out"=w308:errorcluster)  [unwired: 8 in]
      }
      frame "Software Reset" {
        n126 = for {
          N: 3 -> [_]
          tunnel: w344 -> [w371]
          tunnel: [w369] -> w347
          n127 = Unbundle By Name(w371) -> ("NFC _Serial.COM"=w370:refnum<visa-resource-name>)
          n128 = call "NFC_Connect.vi"("VISA resource name"=w370) -> ("NFC"=w369:bool)  [unwired: 9 in, 1 out]
        }
        n129 = case shown="真" w347 {
          tunnel: w343 -> [_ w365]
          tunnel: w342 -> [_ w362]
          tunnel: ["UUT Sleep" w357] -> w341
          frame False {
          }
          frame True {
            n130 = Build Path(base path=w365, name or relative path=w362) -> (appended path=w366:path)
            n131 = call "SendCmd_Tool.vi"("path_bat"=w366) -> ("return code"=w364:i32)  [unwired: 7 in, 7 out]
            n132 = call "NFC_Result.vi"("return code"=w364) -> ("return_result"=w363:string)  [unwired: 9 in, 1 out]
            n133 = call <vilib>:"Trim Whitespace.vi"("string"=w363) -> ("trimmed string"=w361:string)  [unwired: 1 in]
            n134 = Concatenate Strings(w361, "   ", w362) -> (w358:string)
            n135 = flat-sequence {
              tunnel: u32 10000 ("milliseconds to wait") -> [w368]
              tunnel: w358 -> [w367]
              tunnel: [w367] -> w357
              frame #0 {
                n136 = Wait (ms)(milliseconds to wait=w368) -> ()  [unwired: 1 out]
              }
            }
          }
        }
        n137 = call "SW_Config.vi"("Step"=enum16{"Initial", "Write", "Read"}."Read") -> ("SW Config out"=w335:T8)  [unwired: 9 in, 1 out]
        n138 = Unbundle By Name(w335) -> ("682_Tool_Repeat"=w334:string)
        n139 = property on="Numeric" class="DigNum (严格)"() -> ("Value"=w340:i32)  [unwired: 2 in, 2 out]
        n140 = Decimal String To Number(string=w334) -> (number=w333:i32)  [unwired: 2 in, 1 out]
        n141 = Increment(x=w340) -> (x+1=w339:i32)
        n142 = Decrement(x=w333) -> (x-1=w332:i32)
        n143 = Greater Or Equal?(x=w339, y=w332) -> (x >= y?=→"Reflect_Flag":bool)
        n144 = property on="Numeric" class="DigNum (严格)"("Value"=w339) -> ()  [unwired: 2 in, 2 out]
        n145 = Concatenate Strings(w351, w348, w341) -> (w352:string)
        n146 = Not(x=w347) -> (.not. x?=w338:bool)
        n147 = call "LogStatus.vi"("error in (no error)"=w349, "last message"=w353, "message"=w352) -> ("error  out"=w354:errorcluster)  [unwired: 8 in]
      }
      frame "Software Reset_once" {
        n148 = for {
          N: 3 -> [_]
          tunnel: w377 -> [w403]
          tunnel: [w401] -> w379
          n149 = Unbundle By Name(w403) -> ("NFC _Serial.COM"=w402:refnum<visa-resource-name>)
          n150 = call "NFC_Connect.vi"("VISA resource name"=w402) -> ("NFC"=w401:bool)  [unwired: 9 in, 1 out]
        }
        n151 = case shown="真" w379 {
          tunnel: w376 -> [_ w397]
          tunnel: w375 -> [_ w394]
          tunnel: ["UUT Sleep" w389] -> w374
          frame False {
          }
          frame True {
            n152 = Build Path(base path=w397, name or relative path=w394) -> (appended path=w398:path)
            n153 = call "SendCmd_Tool.vi"("path_bat"=w398) -> ("return code"=w396:i32)  [unwired: 7 in, 7 out]
            n154 = call "NFC_Result.vi"("return code"=w396) -> ("return_result"=w395:string)  [unwired: 9 in, 1 out]
            n155 = call <vilib>:"Trim Whitespace.vi"("string"=w395) -> ("trimmed string"=w393:string)  [unwired: 1 in]
            n156 = Concatenate Strings(w393, "   ", w394) -> (w390:string)
            n157 = flat-sequence {
              tunnel: u32 10000 ("milliseconds to wait") -> [w400]
              tunnel: w390 -> [w399]
              tunnel: [w399] -> w389
              frame #0 {
                n158 = Wait (ms)(milliseconds to wait=w400) -> ()  [unwired: 1 out]
              }
            }
          }
        }
        n159 = Concatenate Strings(w383, w380, w374) -> (w384:string)
        n160 = Not(x=w379) -> (.not. x?=w373:bool)
        n161 = call "LogStatus.vi"("error in (no error)"=w381, "last message"=w385, "message"=w384) -> ("error  out"=w386:errorcluster)  [unwired: 8 in]
      }
      frame "Software Reset1" {
        n162 = for {
          N: 3 -> [_]
          tunnel: w416 -> [w443]
          tunnel: [w441] -> w419
          n163 = Unbundle By Name(w443) -> ("NFC _Serial.COM"=w442:refnum<visa-resource-name>)
          n164 = call "NFC_Connect.vi"("VISA resource name"=w442) -> ("NFC"=w441:bool)  [unwired: 9 in, 1 out]
        }
        n165 = case shown="真" w419 {
          tunnel: w415 -> [_ w437]
          tunnel: w414 -> [_ w434]
          tunnel: ["UUT Sleep" w429] -> w413
          frame False {
          }
          frame True {
            n166 = Build Path(base path=w437, name or relative path=w434) -> (appended path=w438:path)
            n167 = call "SendCmd_Tool.vi"("path_bat"=w438) -> ("return code"=w436:i32)  [unwired: 7 in, 7 out]
            n168 = call "NFC_Result.vi"("return code"=w436) -> ("return_result"=w435:string)  [unwired: 9 in, 1 out]
            n169 = call <vilib>:"Trim Whitespace.vi"("string"=w435) -> ("trimmed string"=w433:string)  [unwired: 1 in]
            n170 = Concatenate Strings(w433, "   ", w434) -> (w430:string)
            n171 = flat-sequence {
              tunnel: u32 10000 ("milliseconds to wait") -> [w440]
              tunnel: w430 -> [w439]
              tunnel: [w439] -> w429
              frame #0 {
                n172 = Wait (ms)(milliseconds to wait=w440) -> ()  [unwired: 1 out]
              }
            }
          }
        }
        n173 = call "SW_Config.vi"("Step"=enum16{"Initial", "Write", "Read"}."Read") -> ("SW Config out"=w408:T8)  [unwired: 9 in, 1 out]
        n174 = Unbundle By Name(w408) -> ("682_Tool_Repeat"=w407:string)
        n175 = property on="Numeric 2" class="DigNum (严格)"() -> ("Value"=w411:i32)  [unwired: 2 in, 2 out]
        n176 = Increment(x=w411) -> (x+1=w404:i32)
        n177 = Decimal String To Number(string=w407) -> (number=w406:i32)  [unwired: 2 in, 1 out]
        n178 = Decrement(x=w406) -> (x-1=w405:i32)
        n179 = Greater Or Equal?(x=w404, y=w405) -> (x >= y?=→"Unifority_Flag":bool)
        n180 = property on="Numeric 2" class="DigNum (严格)"("Value"=w404) -> ()  [unwired: 2 in, 2 out]
        n181 = Concatenate Strings(w423, w420, w413) -> (w424:string)
        n182 = Not(x=w419) -> (.not. x?=w412:bool)
        n183 = call "LogStatus.vi"("error in (no error)"=w421, "last message"=w425, "message"=w424) -> ("error  out"=w426:errorcluster)  [unwired: 8 in]
      }
      frame "5.2.3_8 Check Test item Reflection result" {
        n184 = Unbundle By Name(w459) -> ("Table"=w468:string[][], "OK/NG"=w460:bool)
        n185 = Build Path(base path=w452, name or relative path=w456) -> (appended path=w462:path)
        n186 = call "SendCmd_Tool.vi"("path_bat"=w462) -> ("VQT"=w453:string, "return code"=w461:i32)  [unwired: 7 in, 6 out]
        n187 = call "Select_Table_Vaule Enable_Disable.vi"("Action"=w467, "Table"=w468) -> ("Enable"=w466:bool)  [unwired: 8 in, 1 out]
        n188 = Build Path(base path=w452, name or relative path="Reflection_Result") -> (appended path=w450:path)
        n189 = Build Path(base path=w450, name or relative path="test_report.txt") -> (appended path=w448:path)
        n190 = case shown="真" w466 {
          tunnel: [w476 w492] -> w469
          tunnel: w468 -> [w478 w503]
          tunnel: w467 -> [w477 w502]
          tunnel: w465 -> [_ _]
          tunnel: [w474 w484] -> w455
          tunnel: w461 -> [_ w499]
          tunnel: w460 -> [w475 w497]
          tunnel: [w475 w495] -> w458
          tunnel: w456 -> [_ w494]
          tunnel: w453 -> [_ w483]
          tunnel: w448 -> [_ w489]
          tunnel: [_ w486] -> w447
          tunnel: [w474 w485] -> w444
          frame False {
            w482 = "UIdisplay" ("Process (\"\" - local)")
            w476 = "Skip" ("Action")
            w474 = TRUE ("Result")
            n191 = call "Select_Table_Vaule.vi"("Vaule"=w476, "Action"=w477, "Table"=w478) -> ("vaule"=w479:string[])  [unwired: 7 in, 1 out]
            n192 = Build Array (concatenate)(w479, w476, w476) -> (w481:string[])
            n193 = Flatten To XML(anything=w481) -> (xml string=w480:string)
            n194 = call "AMC Send Local Message.vi"("Process (\"\" - local)"=w482, "Message Value"=w480, "Message Name"=w482) -> ()  [unwired: 7 in, 2 out]
          }
          frame True {
            w490 = "   "
            # "TBD"
            n195 = call "NFC_Result.vi"("input"=w483, "return code"=w499) -> ("Command Sucess"=w484:bool, "return_result"=w500:string)  [unwired: 8 in]
            n196 = Select(t=w490, s=w484, f=w483) -> (s? t:f=w491:string)
            n197 = call <vilib>:"Trim Whitespace.vi"("string"=w500) -> ("trimmed string"=w493:string)  [unwired: 1 in]
            n198 = Concatenate Strings(w494, w490, w493, w490, w491) -> (w492:string)
            n199 = case shown="真" w484 {
              tunnel: w489 -> [_ w514]
              tunnel: [FALSE ("Result") w513] -> w487
              tunnel: [_ w512] -> w486
              frame False {
              }
              frame True {
                n200 = call "VOT_Reflect&Unifority.vi"("file (use dialog)"=w514) -> ("Reflect"=w512:string, "Result"=w513:bool)  [unwired: 8 in, 1 out]
              }
            }
            n201 = call "Select_Table_Vaule.vi"("Vaule"=w492, "Action"=w502, "Table"=w503) -> ("Result"=w498:bool, "vaule"=w508:string[])  [unwired: 7 in]
            n202 = And(x=w498, y=w487) -> (x .and. y?=w496:bool)
            n203 = Append True/False String(1:w496, 2:"FAIL" ("真字符串"), 3:"PASS" ("真字符串")) -> (0:w501:string)  [unwired: 1 in]
            n204 = And(x=w497, y=w496) -> (x .and. y?=w495:bool)
            n205 = property on="Reflect_Flag" class="Bool (严格)"() -> ("Value"=w488:bool)  [unwired: 2 in, 2 out]
            n206 = Build Array (concatenate)(w508, w486, w501) -> (w507:string[])
            n207 = Flatten To XML(anything=w507) -> (xml string=w506:string)
            n208 = Or(x=w488, y=w484) -> (x .or. y?=w485:bool)
            n209 = case shown="真" w485 {
              tunnel: w506 -> [_ w509]
              frame False {
              }
              frame True {
                w510 = "UIdisplay" ("Process (\"\" - local)")
                n210 = call "AMC Send Local Message.vi"("Process (\"\" - local)"=w510, "Message Value"=w509, "Message Name"=w510) -> ()  [unwired: 7 in, 2 out]
              }
            }
          }
        }
        n211 = Concatenate Strings(w467, w463, w469) -> (w470:string)
        n212 = Bundle By Name(cluster=w459, "OK/NG"=w458, "VOT.Reflection"=w447) -> (w457:T2)
        n213 = call "LogStatus.vi"("error in (no error)"=w464, "last message"=w471, "message"=w470) -> ("error  out"=w472:errorcluster)  [unwired: 8 in]
        n214 = Select(t=w445, s=w444, f="Software Reset") -> (s? t:f=w446:string)
        n215 = call "FailResumeMode.vi"("OK/NG"=w455, "EndMessage"=w445) -> ()  [unwired: 7 in, 1 out]
      }
      frame "5.2.3_10 VQT_Uniformity_Initial brightness" {
        n216 = Unbundle By Name(w534) -> ("Table"=w545:string[][], "OK/NG"=w536:bool)
        n217 = Build Path(base path=w524, name or relative path=w528) -> (appended path=w538:path)
        n218 = call "SendCmd_Tool.vi"("path_bat"=w538) -> ("VQT"=w529:string, "return code"=w537:i32)  [unwired: 7 in, 6 out]
        n219 = call "Select_Table_Vaule Enable_Disable.vi"("Action"=w544, "Table"=w545) -> ("Enable"=w543:bool)  [unwired: 8 in, 1 out]
        n220 = Build Path(base path=w524, name or relative path="Uniformity_Result") -> (appended path=w526:path)
        n221 = Build Path(base path=w526, name or relative path="test_report.txt") -> (appended path=w523:path)
        n222 = case shown="真" w543 {
          tunnel: [w553 w568] -> w546
          tunnel: w545 -> [w555 w588]
          tunnel: w544 -> [w554 w587]
          tunnel: w542 -> [_ _]
          tunnel: [TRUE ("Result") w563] -> w530
          tunnel: w537 -> [_ w584]
          tunnel: w536 -> [w552 w582]
          tunnel: [w552 w581] -> w535
          tunnel: w529 -> [_ w578]
          tunnel: w528 -> [_ w580]
          tunnel: w523 -> [_ w575]
          tunnel: [_ w564] -> w522
          tunnel: [_ w572] -> w521
          tunnel: [_ w571] -> w520
          tunnel: [_ w570] -> w519
          tunnel: [_ w567] -> w518
          tunnel: [_ w569] -> w517
          tunnel: [FALSE w561] -> w516
          frame False {
            w559 = "UIdisplay" ("Process (\"\" - local)")
            w553 = "Skip" ("Action")
            n223 = call "Select_Table_Vaule.vi"("Vaule"=w553, "Action"=w554, "Table"=w555) -> ("vaule"=w556:string[])  [unwired: 7 in, 1 out]
            n224 = Build Array (concatenate)(w556, w553, w553) -> (w558:string[])
            n225 = Flatten To XML(anything=w558) -> (xml string=w557:string)
            n226 = call "AMC Send Local Message.vi"("Process (\"\" - local)"=w559, "Message Value"=w557, "Message Name"=w559) -> ()  [unwired: 7 in, 2 out]
          }
          frame True {
            w577 = "   "
            n227 = call "NFC_Result.vi"("input"=w578, "return code"=w584) -> ("Command Sucess"=w562:bool, "return_result"=w585:string)  [unwired: 8 in]
            n228 = call <vilib>:"Trim Whitespace.vi"("string"=w585) -> ("trimmed string"=w579:string)  [unwired: 1 in]
            n229 = Select(t=w577, s=w562, f=w578) -> (s? t:f=w576:string)
            n230 = case shown="真" w562 {
              tunnel: w575 -> [_ w599]
              tunnel: [_ w598] -> w574
              tunnel: [FALSE ("Result") w597] -> w565
              frame False {
              }
              frame True {
                n231 = call "VOT_Reflect&Unifority.vi"("file (use dialog)"=w599) -> ("Unifority"=w598:string[], "Result"=w597:bool)  [unwired: 8 in, 1 out]
              }
            }
            n232 = Concatenate Strings(w580, w577, w579, w577, w576) -> (w568:string)
            n233 = call "Select_Table_Vaule.vi"("Vaule"=w568, "Action"=w587, "Table"=w588) -> ("Result"=w583:bool, "vaule"=w593:string[])  [unwired: 7 in]
            n234 = And(x=w583, y=w565) -> (x .and. y?=w561:bool)
            n235 = Index Array(array=w574, index #1=0 ("index")) -> (element #1=w564:string, element #2=w572:string, element #3=w571:string, element #4=w570:string, element #5=w567:string, element #6=w569:string)  [unwired: 5 in]
            n236 = Append True/False String(1:w561, 2:"FAIL" ("真字符串"), 3:"PASS" ("真字符串")) -> (0:w586:string)  [unwired: 1 in]
            n237 = And(x=w561, y=w582) -> (x .and. y?=w581:bool)
            n238 = Build Array (concatenate)(w593, w564, w586) -> (w592:string[])
            n239 = property on="Unifority_Flag" class="Bool (严格)"() -> ("Value"=w566:bool)  [unwired: 2 in, 2 out]
            n240 = Flatten To XML(anything=w592) -> (xml string=w591:string)
            n241 = Or(x=w566, y=w562) -> (x .or. y?=w563:bool)
            n242 = case shown="真" w563 {
              tunnel: w591 -> [_ w594]
              frame False {
              }
              frame True {
                w595 = "UIdisplay" ("Process (\"\" - local)")
                n243 = call "AMC Send Local Message.vi"("Process (\"\" - local)"=w595, "Message Value"=w594, "Message Name"=w595) -> ()  [unwired: 7 in, 2 out]
              }
            }
          }
        }
        n244 = Concatenate Strings(w544, w540, w546) -> (w547:string)
        n245 = Bundle By Name(cluster=w534, "OK/NG"=w535, "VOT.Initial brightness"=w522, "VOT.Mean uniformity"=w521, "VOT.Uniformity_Deviation"=w520, "VOT.Adjusted brightness"=w519, "VOT.Mean_Adjusted"=w518, "VOT.Deviation_Adjusted"=w517, "VOT.Result"=w516) -> (w533:T2)
        n246 = call "LogStatus.vi"("error in (no error)"=w541, "last message"=w548, "message"=w547) -> ("error  out"=w549:errorcluster)  [unwired: 8 in]
        n247 = Select(t="5.2.3_11 VQT_Uniformity_Mean uniformity", s=w530, f="Software Reset1") -> (s? t:f=w515:string)
        n248 = call "FailResumeMode.vi"("OK/NG"=w530, "EndMessage"=w539) -> ()  [unwired: 7 in, 1 out]
      }
      frame "5.2.3_11 VQT_Uniformity_Mean uniformity" {
        n249 = Unbundle By Name(w605) -> ("Table"=w612:string[][], "OK/NG"=w606:bool, "VOT.Mean uniformity"=w602:string, "VOT.Result"=w600:bool)
        n250 = call "Select_Table_Vaule Enable_Disable.vi"("Action"=w611, "Table"=w612) -> ("Enable"=w610:bool)  [unwired: 8 in, 1 out]
        n251 = case shown="真" w610 {
          tunnel: [w619 w627] -> w613
          tunnel: w612 -> [w621 w634]
          tunnel: w611 -> [w620 w633]
          tunnel: w609 -> [_ _]
          tunnel: w606 -> [w618 w631]
          tunnel: [w618 w628] -> w604
          tunnel: w602 -> [_ w627]
          tunnel: w600 -> [_ w626]
          frame False {
            w625 = "UIdisplay" ("Process (\"\" - local)")
            w619 = "Skip" ("Action")
            n252 = call "Select_Table_Vaule.vi"("Vaule"=w619, "Action"=w620, "Table"=w621) -> ("vaule"=w622:string[])  [unwired: 7 in, 1 out]
            n253 = Build Array (concatenate)(w622, w619, w619) -> (w624:string[])
            n254 = Flatten To XML(anything=w624) -> (xml string=w623:string)
            n255 = call "AMC Send Local Message.vi"("Process (\"\" - local)"=w625, "Message Value"=w623, "Message Name"=w625) -> ()  [unwired: 7 in, 2 out]
          }
          frame True {
            w639 = "UIdisplay" ("Process (\"\" - local)")
            n256 = call "Select_Table_Vaule.vi"("Vaule"=w627, "Action"=w633, "Table"=w634) -> ("Result"=w630:bool, "vaule"=w640:string[])  [unwired: 7 in]
            n257 = And(x=w626, y=w630) -> (x .and. y?=w629:bool)
            n258 = Append True/False String(1:w629, 2:"FAIL" ("真字符串"), 3:"PASS" ("真字符串")) -> (0:w632:string)  [unwired: 1 in]
            n259 = Build Array (concatenate)(w640, w627, w632) -> (w638:string[])
            n260 = And(x=w631, y=w629) -> (x .and. y?=w628:bool)
            n261 = Flatten To XML(anything=w638) -> (xml string=w637:string)
            n262 = call "AMC Send Local Message.vi"("Process (\"\" - local)"=w639, "Message Value"=w637, "Message Name"=w639) -> ()  [unwired: 7 in, 2 out]
          }
        }
        n263 = Concatenate Strings(w611, w607, w613) -> (w614:string)
        n264 = call "LogStatus.vi"("error in (no error)"=w608, "last message"=w615, "message"=w614) -> ("error  out"=w616:errorcluster)  [unwired: 8 in]
        n265 = Bundle By Name(cluster=w605, "OK/NG"=w604) -> (w603:T2)
      }
      frame "5.2.3_12 VQT_Uniformity_Deviation" {
        n266 = Unbundle By Name(w646) -> ("Table"=w653:string[][], "OK/NG"=w647:bool, "VOT.Uniformity_Deviation"=w643:string, "VOT.Result"=w641:bool)
        n267 = call "Select_Table_Vaule Enable_Disable.vi"("Action"=w652, "Table"=w653) -> ("Enable"=w651:bool)  [unwired: 8 in, 1 out]
        n268 = case shown="真" w651 {
          tunnel: [w661 w668] -> w654
          tunnel: w653 -> [w662 w675]
          tunnel: w652 -> [w660 w674]
          tunnel: w650 -> [_ _]
          tunnel: w647 -> [w659 w672]
          tunnel: [w659 w669] -> w645
          tunnel: w643 -> [_ w668]
          tunnel: w641 -> [_ w667]
          frame False {
            w666 = "UIdisplay" ("Process (\"\" - local)")
            w661 = "Skip" ("Action")
            n269 = call "Select_Table_Vaule.vi"("Vaule"=w661, "Action"=w660, "Table"=w662) -> ("vaule"=w663:string[])  [unwired: 7 in, 1 out]
            n270 = Build Array (concatenate)(w663, w661, w661) -> (w665:string[])
            n271 = Flatten To XML(anything=w665) -> (xml string=w664:string)
            n272 = call "AMC Send Local Message.vi"("Process (\"\" - local)"=w666, "Message Value"=w664, "Message Name"=w666) -> ()  [unwired: 7 in, 2 out]
          }
          frame True {
            w680 = "UIdisplay" ("Process (\"\" - local)")
            n273 = call "Select_Table_Vaule.vi"("Vaule"=w668, "Action"=w674, "Table"=w675) -> ("Result"=w671:bool, "vaule"=w681:string[])  [unwired: 7 in]
            n274 = And(x=w667, y=w671) -> (x .and. y?=w670:bool)
            n275 = Append True/False String(1:w670, 2:"FAIL" ("真字符串"), 3:"PASS" ("真字符串")) -> (0:w673:string)  [unwired: 1 in]
            n276 = Build Array (concatenate)(w681, w668, w673) -> (w679:string[])
            n277 = And(x=w672, y=w670) -> (x .and. y?=w669:bool)
            n278 = Flatten To XML(anything=w679) -> (xml string=w678:string)
            n279 = call "AMC Send Local Message.vi"("Process (\"\" - local)"=w680, "Message Value"=w678, "Message Name"=w680) -> ()  [unwired: 7 in, 2 out]
          }
        }
        n280 = Concatenate Strings(w652, w648, w654) -> (w655:string)
        n281 = call "LogStatus.vi"("error in (no error)"=w649, "last message"=w656, "message"=w655) -> ("error  out"=w657:errorcluster)  [unwired: 8 in]
        n282 = Bundle By Name(cluster=w646, "OK/NG"=w645) -> (w644:T2)
      }
      frame "5.2.3_13 VQT_Uniformity_Adjusted brightness" {
        n283 = Unbundle By Name(w687) -> ("Table"=w694:string[][], "OK/NG"=w688:bool, "VOT.Adjusted brightness"=w684:string, "VOT.Result"=w682:bool)
        n284 = call "Select_Table_Vaule Enable_Disable.vi"("Action"=w693, "Table"=w694) -> ("Enable"=w692:bool)  [unwired: 8 in, 1 out]
        n285 = case shown="真" w692 {
          tunnel: [w701 w709] -> w695
          tunnel: w694 -> [w703 w716]
          tunnel: w693 -> [w702 w715]
          tunnel: w691 -> [_ _]
          tunnel: w688 -> [w700 w713]
          tunnel: [w700 w710] -> w686
          tunnel: w684 -> [_ w709]
          tunnel: w682 -> [_ w708]
          frame False {
            w707 = "UIdisplay" ("Process (\"\" - local)")
            w701 = "Skip" ("Action")
            n286 = call "Select_Table_Vaule.vi"("Vaule"=w701, "Action"=w702, "Table"=w703) -> ("vaule"=w704:string[])  [unwired: 7 in, 1 out]
            n287 = Build Array (concatenate)(w704, w701, w701) -> (w706:string[])
            n288 = Flatten To XML(anything=w706) -> (xml string=w705:string)
            n289 = call "AMC Send Local Message.vi"("Process (\"\" - local)"=w707, "Message Value"=w705, "Message Name"=w707) -> ()  [unwired: 7 in, 2 out]
          }
          frame True {
            w721 = "UIdisplay" ("Process (\"\" - local)")
            n290 = call "Select_Table_Vaule.vi"("Vaule"=w709, "Action"=w715, "Table"=w716) -> ("Result"=w712:bool, "vaule"=w722:string[])  [unwired: 7 in]
            n291 = And(x=w708, y=w712) -> (x .and. y?=w711:bool)
            n292 = Append True/False String(1:w711, 2:"FAIL" ("真字符串"), 3:"PASS" ("真字符串")) -> (0:w714:string)  [unwired: 1 in]
            n293 = Build Array (concatenate)(w722, w709, w714) -> (w720:string[])
            n294 = And(x=w713, y=w711) -> (x .and. y?=w710:bool)
            n295 = Flatten To XML(anything=w720) -> (xml string=w719:string)
            n296 = call "AMC Send Local Message.vi"("Process (\"\" - local)"=w721, "Message Value"=w719, "Message Name"=w721) -> ()  [unwired: 7 in, 2 out]
          }
        }
        n297 = Concatenate Strings(w693, w689, w695) -> (w696:string)
        n298 = call "LogStatus.vi"("error in (no error)"=w690, "last message"=w697, "message"=w696) -> ("error  out"=w698:errorcluster)  [unwired: 8 in]
        n299 = Bundle By Name(cluster=w687, "OK/NG"=w686) -> (w685:T2)
      }
      frame "5.2.3_14 VQT_Uniformity_Mean uniformity" {
        n300 = Unbundle By Name(w728) -> ("Table"=w735:string[][], "OK/NG"=w729:bool, "VOT.Mean_Adjusted"=w725:string, "VOT.Result"=w723:bool)
        n301 = call "Select_Table_Vaule Enable_Disable.vi"("Action"=w734, "Table"=w735) -> ("Enable"=w733:bool)  [unwired: 8 in, 1 out]
        n302 = case shown="真" w733 {
          tunnel: [w742 w750] -> w736
          tunnel: w735 -> [w743 w757]
          tunnel: w734 -> [w742 w756]
          tunnel: w732 -> [_ _]
          tunnel: w729 -> [w741 w754]
          tunnel: [w741 w751] -> w727
          tunnel: w725 -> [_ w750]
          tunnel: w723 -> [_ w749]
          frame False {
            w748 = "UIdisplay" ("Process (\"\" - local)")
            w744 = "Skip" ("Action")
            n303 = call "Select_Table_Vaule.vi"("Vaule"=w744, "Action"=w742, "Table"=w743) -> ("vaule"=w745:string[])  [unwired: 7 in, 1 out]
            n304 = Build Array (concatenate)(w745, w744, w744) -> (w747:string[])
            n305 = Flatten To XML(anything=w747) -> (xml string=w746:string)
            n306 = call "AMC Send Local Message.vi"("Process (\"\" - local)"=w748, "Message Value"=w746, "Message Name"=w748) -> ()  [unwired: 7 in, 2 out]
          }
          frame True {
            w762 = "UIdisplay" ("Process (\"\" - local)")
            n307 = call "Select_Table_Vaule.vi"("Vaule"=w750, "Action"=w756, "Table"=w757) -> ("Result"=w753:bool, "vaule"=w763:string[])  [unwired: 7 in]
            n308 = And(x=w749, y=w753) -> (x .and. y?=w752:bool)
            n309 = Append True/False String(1:w752, 2:"FAIL" ("真字符串"), 3:"PASS" ("真字符串")) -> (0:w755:string)  [unwired: 1 in]
            n310 = Build Array (concatenate)(w763, w750, w755) -> (w761:string[])
            n311 = And(x=w754, y=w752) -> (x .and. y?=w751:bool)
            n312 = Flatten To XML(anything=w761) -> (xml string=w760:string)
            n313 = call "AMC Send Local Message.vi"("Process (\"\" - local)"=w762, "Message Value"=w760, "Message Name"=w762) -> ()  [unwired: 7 in, 2 out]
          }
        }
        n314 = Concatenate Strings(w734, w730, w736) -> (w737:string)
        n315 = call "LogStatus.vi"("error in (no error)"=w731, "last message"=w738, "message"=w737) -> ("error  out"=w739:errorcluster)  [unwired: 8 in]
        n316 = Bundle By Name(cluster=w728, "OK/NG"=w727) -> (w726:T2)
      }
      frame "5.2.3_15 VQT_Uniformity_Deviation" {
        n317 = Unbundle By Name(w769) -> ("Table"=w776:string[][], "OK/NG"=w770:bool, "VOT.Deviation_Adjusted"=w766:string, "VOT.Result"=w764:bool)
        n318 = call "Select_Table_Vaule Enable_Disable.vi"("Action"=w775, "Table"=w776) -> ("Enable"=w774:bool)  [unwired: 8 in, 1 out]
        n319 = case shown="真" w774 {
          tunnel: [w783 w792] -> w777
          tunnel: w776 -> [w785 w798]
          tunnel: w775 -> [w784 w797]
          tunnel: w773 -> [_ _]
          tunnel: w770 -> [w782 w795]
          tunnel: [w782 w793] -> w768
          tunnel: w766 -> [_ w792]
          tunnel: w764 -> [_ w791]
          frame False {
            w789 = "UIdisplay" ("Process (\"\" - local)")
            w783 = "Skip" ("Action")
            n320 = call "Select_Table_Vaule.vi"("Vaule"=w783, "Action"=w784, "Table"=w785) -> ("vaule"=w786:string[])  [unwired: 7 in, 1 out]
            n321 = Build Array (concatenate)(w786, w783, w783) -> (w788:string[])
            n322 = Flatten To XML(anything=w788) -> (xml string=w787:string)
            n323 = call "AMC Send Local Message.vi"("Process (\"\" - local)"=w789, "Message Value"=w787, "Message Name"=w789) -> ()  [unwired: 7 in, 2 out]
          }
          frame True {
            w803 = "UIdisplay" ("Process (\"\" - local)")
            n324 = call "Select_Table_Vaule.vi"("Vaule"=w792, "Action"=w797, "Table"=w798) -> ("Result"=w794:bool, "vaule"=w804:string[])  [unwired: 7 in]
            n325 = And(x=w791, y=w794) -> (x .and. y?=w790:bool)
            n326 = Append True/False String(1:w790, 2:"FAIL" ("真字符串"), 3:"PASS" ("真字符串")) -> (0:w796:string)  [unwired: 1 in]
            n327 = Build Array (concatenate)(w804, w792, w796) -> (w802:string[])
            n328 = And(x=w795, y=w790) -> (x .and. y?=w793:bool)
            n329 = Flatten To XML(anything=w802) -> (xml string=w801:string)
            n330 = call "AMC Send Local Message.vi"("Process (\"\" - local)"=w803, "Message Value"=w801, "Message Name"=w803) -> ()  [unwired: 7 in, 2 out]
          }
        }
        n331 = Concatenate Strings(w775, w771, w777) -> (w778:string)
        n332 = call "LogStatus.vi"("error in (no error)"=w772, "last message"=w779, "message"=w778) -> ("error  out"=w780:errorcluster)  [unwired: 8 in]
        n333 = Bundle By Name(cluster=w769, "OK/NG"=w768) -> (w767:T2)
      }
    }
    n334 = call "6-AlarmStatus.vi"("Step"=enum16{"Initial", "Write", "Read"}."Read") -> ("AlarmValue Out"=w44:bool[])  [unwired: 9 in, 1 out]
    n335 = call "Stop.vi"("Step"=enum16{"Initial", "Write", "Read"}."Read") -> ("Stop Out"=w52:bool)  [unwired: 9 in, 1 out]
    n336 = call "Exit.vi"("Step"=enum16{"Initial", "Write", "Read"}."Read" ("step")) -> ("Exit Out"=w51:bool)  [unwired: 9 in, 1 out]
    n337 = Or Array Elements(Boolean array=w44) -> (logical OR=w43:bool)
    n338 = Compound Arithmetic op=OR(w50, w52, w51, w43) -> (w49:bool)
    n339 = call "AMC Run Step.vi"("Message Queue In"=w67, "Message Name"=w57, "Message Value"=w55, "error in (no error)"=w62, "Mli/Sig"=FALSE) -> ("Message Queue Out"=w66:T4, "error out"=w61:errorcluster)  [unwired: 13 in]
  }
  "Message Queue Out" <- w24
  "error out" <- w23
  "Data out" <- w21
  n340 = property on="Numeric" class="DigNum (严格)"("Value"=w2) -> ()  [unwired: 2 in, 2 out]
  n341 = property on="Numeric 2" class="DigNum (严格)"("Value"=w2) -> ()  [unwired: 2 in, 2 out]
